vi "002_LinFlowChart.vi"(11 "Queue Ref In":T1={"UI"=refnum, "Message"=refnum, "Data"=refnum, "Caller"=refnum, "Name"="000 Common", "Data Path"=path "", "Class Path"=path "", "SubPanel"=refnum, "Project Name"="", "MNT"="", "Title"="", "Data Source"=refnum, "Queue List"={}, "VI"=refnum, "UE"=refnum}) -> ()   [LabVIEW 2020]
doc: "002_LinFlowChart.vi"
uses:
  Alin/QMH/000 Module Data Type.ctl
  Alin/QMH/Queue Message.ctl
  <vilib>/Utility/miscctls.llb/LVPoint32TypeDef.ctl
  <vilib>/Utility/miscctls.llb/LVBoundsTypeDef.ctl
  <vilib>/Utility/miscctls.llb/LVMapReplaceAction.ctl
  <vilib>/Utility/miscctls.llb/LVPositionTypeDef.ctl
  544e2817-58be-4d71-9deb-2b826c4f9655.vi
  <vilib>/Utility/config.llb/Read Key (String).vi
  <vilib>/Utility/file.llb/Read Delimited Spreadsheet (string).vi
  <vilib>/Utility/config.llb/Write Key (String).vi
  <vilib>/Utility/file.llb/Write Delimited Spreadsheet (string).vi
  <vilib>/Utility/config.llb/NI_LVConfig.lvlib
panel:
  in  "ShowLable":bool
  in  "WorkMode Edit":bool
  in  "Load Picture":bool
  in  "FlowChartEdit":bool
  in  "Picture Delete":bool
  in  "Picture Add":bool
  in  "Chart Select":u16(ring) items=["气路", "水路"]
  in  "LogRead":bool
  in  "Panel Show":bool
  in  "FlowChart":T2={"Bump 1"=FALSE, "Bump 2"=FALSE, "LMG 1"=FALSE, "LMG 2"=FALSE, "Data 1"="0", "Data 2"="0", "VValve 1"=FALSE, "HValve 1"=FALSE, "HValve 2"=FALSE, "VValve 2"=FALSE, "HFS 1"=FALSE, "VFS 1"=FALSE, "VFS 2"=FALSE, "HFS 2"=FALSE, "Data 3"="0", "Data 4"="0", "Data 5"="0", "Data 6"="0", "Data 7"="0", "Data 8"="0", "Data 9"="0", "Data 10"="0", "Data 11"="0", "Data 12"="0", "Data 13"="0", "Data 14"="0", "Data 15"="0", "Data 16"="0", "Data 17"="0", "Data 18"="0", "Data 19"="0", "Data 20"="0", "Data 21"="0", "Data 22"="0", "Data 23"="0", "Data 24"="0", "Data 25"="0", "Data 26"="0", "Data 27"="0", "Data 28"="0", "Data 29"="0", "Data 30"="0", "Data 31"="0", "Data 32"="0", "Data 33"="0", "Data 34"="0", "Data 35"="0", "Data 36"="0", "Data 37"="0", "Data 38"="0", "Data 39"="0", "Data 40"="0", "Data 41"="0", "Data 42"="0", "Data 43"="0", "Data 44"="0", "Data 45"="0", "Data 46"="0", "Data 47"="0", "Data 48"="0", "Data 49"="0", "Data 50"="0", "Data 51"="0", "Data 52"="0", "Data 53"="0", "Data 54"="0", "Data 55"="0", "Data 56"="0", "Data 57"="0", "Data 58"="0", "Data 59"="0", "Data 60"="0", "Data 61"="0", "Data 62"="0", "Data 63"="0", "Data 64"="0", "Data 65"="0", "Data 66"="0", "Data 67"="0", "Data 68"="0", "Data 69"="0", "Data 70"="0", "Data 71"="0", "Data 72"="0", "Data 73"="0", "Data 74"="0", "Data 75"="0", "Data 76"="0", "Data 77"="0", "Data 78"="0", "Data 79"="0", "Data 80"="0", "Data 81"="0", "Data 82"="0", "Data 83"="0", "Data 84"="0", "Data 85"="0", "Data 86"="0", "Data 87"="0", "Data 88"="0", "Data 89"="0", "Data 90"="0", "Data 91"="0", "Data 92"="0", "Data 93"="0", "Data 94"="0", "Data 95"="0", "Data 96"="0", "Data 97"="0", "Data 98"="0", "Data 99"="0", "Data 100"="0", "Data 101"="0", "Data 102"="0", "Data 103"="0", "Data 104"="0", "Data 105"="0", "Data 106"="0", "Data 107"="0", "Data 108"="0", "Data 109"="0", "Data 110"="0", "Data 111"="0", "Data 112"="0", "Data 113"="0", "Data 114"="0", "Data 115"="0", "Data 116"="0", "Data 117"="0", "Data 118"="0", "Data 119"="0", "Data 120"="0", "Data 121"="0", "Data 122"="0", "Data 123"="0", "Data 124"="0", "Data 125"="0", "Data 126"="0", "Data 127"="0", "Data 128"="0", "Data 129"="0", "Data 130"="0", "Data 131"="0", "Data 132"="0", "Data 133"="0", "Data 134"="0", "Data 135"="0", "Data 136"="0", "Data 137"="0", "Data 138"="0", "Data 139"="0", "Data 140"="0", "Data 141"="0", "Data 142"="0", "Data 143"="0", "Data 144"="0", "Data 145"="0", "Data 146"="0", "Data 147"="0", "Data 148"="0", "Data 149"="0", "Data 150"="0", "Data 151"="0", "Data 152"="0", "Data 153"="0", "Data 154"="0", "Data 155"="0", "Data 156"="0", "Data 157"="0", "Data 158"="0", "Data 159"="0", "Data 160"="0", "Data 161"="0", "Data 162"="0", "Data 163"="0", "Data 164"="0", "Data 165"="0", "Data 166"="0", "Data 167"="0", "Data 168"="0", "Data 169"="0", "Data 170"="0", "Data 171"="0", "Data 172"="0", "Data 173"="0", "Data 174"="0", "Data 175"="0", "Data 176"="0", "Data 177"="0", "Data 178"="0", "Data 179"="0", "Data 180"="0", "Data 181"="0", "Data 182"="0", "Data 183"="0", "Data 184"="0", "Data 185"="0", "Data 186"="0", "Data 187"="0", "Data 188"="0", "Data 189"="0", "Data 190"="0", "Data 191"="0", "Data 192"="0", "LMG 3"=FALSE, "LMG 4"=FALSE, "LMG 5"=FALSE, "LMG 6"=FALSE, "LMG 7"=FALSE, "LMG 8"=FALSE, "LMG 9"=FALSE, "LMG 10"=FALSE, "LMG 11"=FALSE, "LMG 12"=FALSE, "LMG 13"=FALSE, "LMG 14"=FALSE, "LMG 15"=FALSE, "LMG 16"=FALSE, "LMG 17"=FALSE, "LMG 18"=FALSE, "LMG 19"=FALSE, "LMG 20"=FALSE, "LMG 21"=FALSE, "LMG 22"=FALSE, "LMG 23"=FALSE, "LMG 24"=FALSE, "LMG 25"=FALSE, "LMG 26"=FALSE, "LMG 27"=FALSE, "LMG 28"=FALSE, "LMG 29"=FALSE, "LMG 30"=FALSE, "LMG 31"=FALSE, "LMG 32"=FALSE, "LMG 33"=FALSE, "LMG 34"=FALSE, "LMG 35"=FALSE, "LMG 36"=FALSE, "LMG 37"=FALSE, "LMG 38"=FALSE, "LMG 39"=FALSE, "LMG 40"=FALSE, "HValve 3"=FALSE, "HValve 4"=FALSE, "HValve 5"=FALSE, "HValve 6"=FALSE, "HValve 7"=FALSE, "HValve 8"=FALSE, "HValve 9"=FALSE, "HValve 10"=FALSE, "HValve 11"=FALSE, "HValve 12"=FALSE, "HValve 13"=FALSE, "HValve 14"=FALSE, "HValve 15"=FALSE, "HValve 16"=FALSE, "HValve 17"=FALSE, "HValve 18"=FALSE, "HValve 19"=FALSE, "HValve 20"=FALSE, "HValve 21"=FALSE, "HValve 22"=FALSE, "HValve 23"=FALSE, "HValve 24"=FALSE, "HValve 25"=FALSE, "HValve 26"=FALSE, "HValve 27"=FALSE, "HValve 28"=FALSE, "HValve 29"=FALSE, "HValve 30"=FALSE, "HValve 31"=FALSE, "HValve 32"=FALSE, "HValve 33"=FALSE, "HValve 34"=FALSE, "HValve 35"=FALSE, "HValve 36"=FALSE, "HValve 37"=FALSE, "HValve 38"=FALSE, "HValve 39"=FALSE, "HValve 40"=FALSE, "HValve 41"=FALSE, "HValve 42"=FALSE, "HValve 43"=FALSE, "HValve 44"=FALSE, "HValve 45"=FALSE, "HValve 46"=FALSE, "HValve 47"=FALSE, "HValve 48"=FALSE, "HValve 49"=FALSE, "HValve 50"=FALSE, "HValve 51"=FALSE, "HValve 52"=FALSE, "HValve 53"=FALSE, "HValve 54"=FALSE, "HValve 55"=FALSE, "HValve 56"=FALSE, "HValve 57"=FALSE, "HValve 58"=FALSE, "HValve 59"=FALSE, "HValve 60"=FALSE, "HValve 61"=FALSE, "HValve 62"=FALSE, "HValve 63"=FALSE, "HValve 64"=FALSE, "HValve 65"=FALSE, "HValve 66"=FALSE, "HValve 67"=FALSE, "HValve 68"=FALSE, "HValve 69"=FALSE, "HValve 70"=FALSE, "HValve 71"=FALSE, "HValve 72"=FALSE, "HValve 73"=FALSE, "HValve 74"=FALSE, "HValve 75"=FALSE, "HValve 76"=FALSE, "HValve 77"=FALSE, "HValve 78"=FALSE, "HValve 79"=FALSE, "HValve 80"=FALSE, "VValve 3"=FALSE, "VValve 4"=FALSE, "VValve 5"=FALSE, "VValve 6"=FALSE, "VValve 7"=FALSE, "VValve 8"=FALSE, "VValve 9"=FALSE, "VValve 10"=FALSE, "VValve 11"=FALSE, "VValve 12"=FALSE, "VValve 13"=FALSE, "VValve 14"=FALSE, "VValve 15"=FALSE, "VValve 16"=FALSE, "VValve 17"=FALSE, "VValve 18"=FALSE, "VValve 19"=FALSE, "VValve 20"=FALSE, "Bump 3"=FALSE, "Bump 4"=FALSE, "Bump 5"=FALSE, "Bump 6"=FALSE, "Bump 7"=FALSE, "Bump 8"=FALSE, "Bump 9"=FALSE, "Bump 10"=FALSE, "VFS 3"=FALSE, "VFS 4"=FALSE, "VFS 5"=FALSE, "VFS 6"=FALSE, "VFS 7"=FALSE, "VFS 8"=FALSE, "VFS 9"=FALSE, "VFS 10"=FALSE, "HFS 3"=FALSE, "HFS 4"=FALSE, "HFS 5"=FALSE, "HFS 6"=FALSE, "HFS 7"=FALSE, "HFS 8"=FALSE, "HFS 9"=FALSE, "HFS 10"=FALSE, "PRT 1"="0", "PRT 2"="0", "PRT 3"="0", "PRT 4"="0", "PRT 5"="0", "PRT 6"="0", "PRT 7"="0", "PRT 8"="0", "PRT 9"="0", "PRT 10"="0", "PRT 11"="0", "PRT 12"="0", "PRT 13"="0", "PRT 14"="0", "PRT 15"="0", "PRT 16"="0", "PRT 17"="0", "PRT 18"="0", "PRT 19"="0", "PRT 20"="0", "HVFS 1"=FALSE, "VVFS 1"=FALSE, "HVFS 2"=FALSE, "HVFS 3"=FALSE, "HVFS 4"=FALSE, "HVFS 5"=FALSE, "HVFS 6"=FALSE, "HVFS 7"=FALSE, "HVFS 8"=FALSE, "HVFS 9"=FALSE, "HVFS 10"=FALSE, "HVFS 11"=FALSE, "HVFS 12"=FALSE, "HVFS 13"=FALSE, "HVFS 14"=FALSE, "HVFS 15"=FALSE, "HVFS 16"=FALSE, "HVFS 17"=FALSE, "HVFS 18"=FALSE, "HVFS 19"=FALSE, "HVFS 20"=FALSE, "VVFS 2"=FALSE, "VVFS 3"=FALSE, "VVFS 4"=FALSE, "VVFS 5"=FALSE, "VVFS 6"=FALSE, "VVFS 7"=FALSE, "VVFS 8"=FALSE, "VVFS 9"=FALSE, "VVFS 10"=FALSE, "VVFS 11"=FALSE, "VVFS 12"=FALSE, "VVFS 13"=FALSE, "VVFS 14"=FALSE, "VVFS 15"=FALSE, "VVFS 16"=FALSE, "VVFS 17"=FALSE, "VVFS 18"=FALSE, "VVFS 19"=FALSE, "VVFS 20"=FALSE, "NHVFS 100"=FALSE, "NVFS 100"=FALSE, "NHFS 100"=FALSE, "NHVFS 101"=FALSE, "NVFS 101"=FALSE, "NHFS 101"=FALSE, "NHVFS 102"=FALSE, "NVFS 102"=FALSE, "NHFS 102"=FALSE, "NHVFS 103"=FALSE, "NVFS 103"=FALSE, "NHFS 103"=FALSE, "NHVFS 104"=FALSE, "NVFS 104"=FALSE, "NHFS 104"=FALSE, "NHVFS 105"=FALSE, "NVFS 105"=FALSE, "NHFS 105"=FALSE, "NHVFS 106"=FALSE, "NVFS 106"=FALSE, "NHFS 106"=FALSE, "NHVFS 107"=FALSE, "NVFS 107"=FALSE, "NHFS 107"=FALSE, "NHVFS 108"=FALSE, "NVFS 108"=FALSE, "NHFS 108"=FALSE, "NHVFS 109"=FALSE, "NVFS 109"=FALSE, "NHFS 109"=FALSE}
  out "Picture":picture
  out "Tips":string
  in  "Decimal":u16=1 max=6
  in  "Horizontal scroll bar":bool caption="H"
  in  "Vertical scroll bar":bool caption="V"
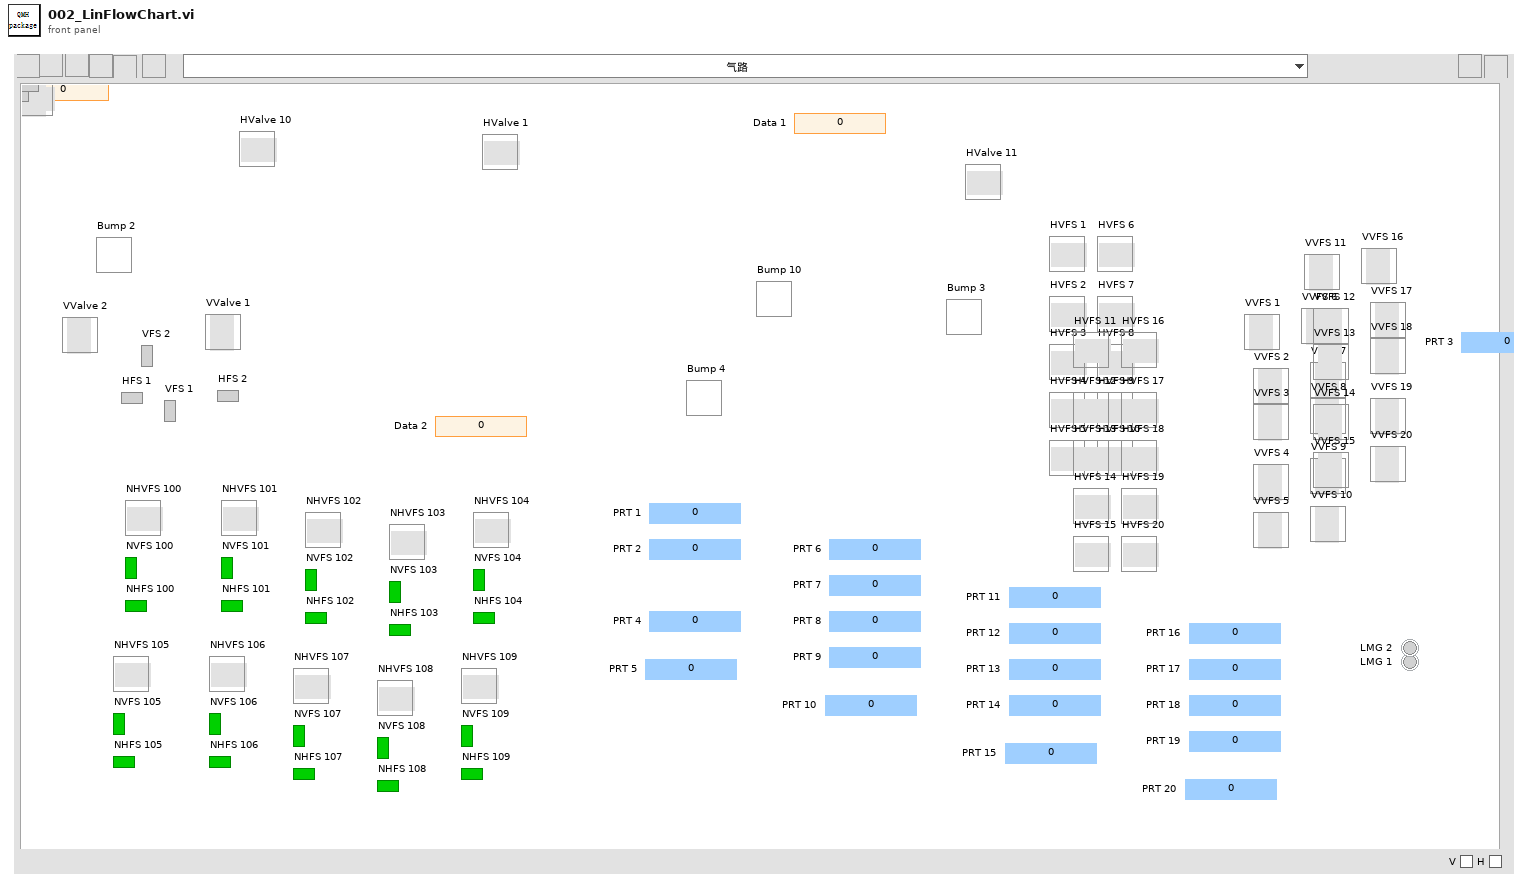
[diagram p1: front panel]
types:
  T1 = typedef "000 Module Data Type.ctl" = cluster{"UI":refnum<queue>, "Message":refnum<queue>, "Data":refnum<queue>, "Caller":refnum<queue>, "Name":string, "Data Path":path, "Class Path":path, "SubPanel":refnum<vi>, "Project Name":string, "MNT":string, "Title":string, "Data Source":refnum<queue>, "Queue List":map{string, refnum<queue>}, "VI":refnum<vi>, "UE":refnum<user-event>}
  T2 = cluster{"Bump 1":bool, "Bump 2":bool, "LMG 1":bool, "LMG 2":bool, "Data 1":string, "Data 2":string, "VValve 1":bool, "HValve 1":bool, "HValve 2":bool, "VValve 2":bool, "HFS 1":bool, "VFS 1":bool, "VFS 2":bool, "HFS 2":bool, "Data 3":string, "Data 4":string, "Data 5":string, "Data 6":string, "Data 7":string, "Data 8":string, "Data 9":string, "Data 10":string, "Data 11":string, "Data 12":string, "Data 13":string, "Data 14":string, "Data 15":string, "Data 16":string, "Data 17":string, "Data 18":string, "Data 19":string, "Data 20":string, "Data 21":string, "Data 22":string, "Data 23":string, "Data 24":string, "Data 25":string, "Data 26":string, "Data 27":string, "Data 28":string, "Data 29":string, "Data 30":string, "Data 31":string, "Data 32":string, "Data 33":string, "Data 34":string, "Data 35":string, "Data 36":string, "Data 37":string, "Data 38":string, "Data 39":string, "Data 40":string, "Data 41":string, "Data 42":string, "Data 43":string, "Data 44":string, "Data 45":string, "Data 46":string, "Data 47":string, "Data 48":string, "Data 49":string, "Data 50":string, "Data 51":string, "Data 52":string, "Data 53":string, "Data 54":string, "Data 55":string, "Data 56":string, "Data 57":string, "Data 58":string, "Data 59":string, "Data 60":string, "Data 61":string, "Data 62":string, "Data 63":string, "Data 64":string, "Data 65":string, "Data 66":string, "Data 67":string, "Data 68":string, "Data 69":string, "Data 70":string, "Data 71":string, "Data 72":string, "Data 73":string, "Data 74":string, "Data 75":string, "Data 76":string, "Data 77":string, "Data 78":string, "Data 79":string, "Data 80":string, "Data 81":string, "Data 82":string, "Data 83":string, "Data 84":string, "Data 85":string, "Data 86":string, "Data 87":string, "Data 88":string, "Data 89":string, "Data 90":string, "Data 91":string, "Data 92":string, "Data 93":string, "Data 94":string, "Data 95":string, "Data 96":string, "Data 97":string, "Data 98":string, "Data 99":string, "Data 100":string, "Data 101":string, "Data 102":string, "Data 103":string, "Data 104":string, "Data 105":string, "Data 106":string, "Data 107":string, "Data 108":string, "Data 109":string, "Data 110":string, "Data 111":string, "Data 112":string, "Data 113":string, "Data 114":string, "Data 115":string, "Data 116":string, "Data 117":string, "Data 118":string, "Data 119":string, "Data 120":string, "Data 121":string, "Data 122":string, "Data 123":string, "Data 124":string, "Data 125":string, "Data 126":string, "Data 127":string, "Data 128":string, "Data 129":string, "Data 130":string, "Data 131":string, "Data 132":string, "Data 133":string, "Data 134":string, "Data 135":string, "Data 136":string, "Data 137":string, "Data 138":string, "Data 139":string, "Data 140":string, "Data 141":string, "Data 142":string, "Data 143":string, "Data 144":string, "Data 145":string, "Data 146":string, "Data 147":string, "Data 148":string, "Data 149":string, "Data 150":string, "Data 151":string, "Data 152":string, "Data 153":string, "Data 154":string, "Data 155":string, "Data 156":string, "Data 157":string, "Data 158":string, "Data 159":string, "Data 160":string, "Data 161":string, "Data 162":string, "Data 163":string, "Data 164":string, "Data 165":string, "Data 166":string, "Data 167":string, "Data 168":string, "Data 169":string, "Data 170":string, "Data 171":string, "Data 172":string, "Data 173":string, "Data 174":string, "Data 175":string, "Data 176":string, "Data 177":string, "Data 178":string, "Data 179":string, "Data 180":string, "Data 181":string, "Data 182":string, "Data 183":string, "Data 184":string, "Data 185":string, "Data 186":string, "Data 187":string, "Data 188":string, "Data 189":string, "Data 190":string, "Data 191":string, "Data 192":string, "LMG 3":bool, "LMG 4":bool, "LMG 5":bool, "LMG 6":bool, "LMG 7":bool, "LMG 8":bool, "LMG 9":bool, "LMG 10":bool, "LMG 11":bool, "LMG 12":bool, "LMG 13":bool, "LMG 14":bool, "LMG 15":bool, "LMG 16":bool, "LMG 17":bool, "LMG 18":bool, "LMG 19":bool, "LMG 20":bool, "LMG 21":bool, "LMG 22":bool, "LMG 23":bool, "LMG 24":bool, "LMG 25":bool, "LMG 26":bool, "LMG 27":bool, "LMG 28":bool, "LMG 29":bool, "LMG 30":bool, "LMG 31":bool, "LMG 32":bool, "LMG 33":bool, "LMG 34":bool, "LMG 35":bool, "LMG 36":bool, "LMG 37":bool, "LMG 38":bool, "LMG 39":bool, "LMG 40":bool, "HValve 3":bool, "HValve 4":bool, "HValve 5":bool, "HValve 6":bool, "HValve 7":bool, "HValve 8":bool, "HValve 9":bool, "HValve 10":bool, "HValve 11":bool, "HValve 12":bool, "HValve 13":bool, "HValve 14":bool, "HValve 15":bool, "HValve 16":bool, "HValve 17":bool, "HValve 18":bool, "HValve 19":bool, "HValve 20":bool, "HValve 21":bool, "HValve 22":bool, "HValve 23":bool, "HValve 24":bool, "HValve 25":bool, "HValve 26":bool, "HValve 27":bool, "HValve 28":bool, "HValve 29":bool, "HValve 30":bool, "HValve 31":bool, "HValve 32":bool, "HValve 33":bool, "HValve 34":bool, "HValve 35":bool, "HValve 36":bool, "HValve 37":bool, "HValve 38":bool, "HValve 39":bool, "HValve 40":bool, "HValve 41":bool, "HValve 42":bool, "HValve 43":bool, "HValve 44":bool, "HValve 45":bool, "HValve 46":bool, "HValve 47":bool, "HValve 48":bool, "HValve 49":bool, "HValve 50":bool, "HValve 51":bool, "HValve 52":bool, "HValve 53":bool, "HValve 54":bool, "HValve 55":bool, "HValve 56":bool, "HValve 57":bool, "HValve 58":bool, "HValve 59":bool, "HValve 60":bool, "HValve 61":bool, "HValve 62":bool, "HValve 63":bool, "HValve 64":bool, "HValve 65":bool, "HValve 66":bool, "HValve 67":bool, "HValve 68":bool, "HValve 69":bool, "HValve 70":bool, "HValve 71":bool, "HValve 72":bool, "HValve 73":bool, "HValve 74":bool, "HValve 75":bool, "HValve 76":bool, "HValve 77":bool, "HValve 78":bool, "HValve 79":bool, "HValve 80":bool, "VValve 3":bool, "VValve 4":bool, "VValve 5":bool, "VValve 6":bool, "VValve 7":bool, "VValve 8":bool, "VValve 9":bool, "VValve 10":bool, "VValve 11":bool, "VValve 12":bool, "VValve 13":bool, "VValve 14":bool, "VValve 15":bool, "VValve 16":bool, "VValve 17":bool, "VValve 18":bool, "VValve 19":bool, "VValve 20":bool, "Bump 3":bool, "Bump 4":bool, "Bump 5":bool, "Bump 6":bool, "Bump 7":bool, "Bump 8":bool, "Bump 9":bool, "Bump 10":bool, "VFS 3":bool, "VFS 4":bool, "VFS 5":bool, "VFS 6":bool, "VFS 7":bool, "VFS 8":bool, "VFS 9":bool, "VFS 10":bool, "HFS 3":bool, "HFS 4":bool, "HFS 5":bool, "HFS 6":bool, "HFS 7":bool, "HFS 8":bool, "HFS 9":bool, "HFS 10":bool, "PRT 1":string, "PRT 2":string, "PRT 3":string, "PRT 4":string, "PRT 5":string, "PRT 6":string, "PRT 7":string, "PRT 8":string, "PRT 9":string, "PRT 10":string, "PRT 11":string, "PRT 12":string, "PRT 13":string, "PRT 14":string, "PRT 15":string, "PRT 16":string, "PRT 17":string, "PRT 18":string, "PRT 19":string, "PRT 20":string, "HVFS 1":bool, "VVFS 1":bool, "HVFS 2":bool, "HVFS 3":bool, "HVFS 4":bool, "HVFS 5":bool, "HVFS 6":bool, "HVFS 7":bool, "HVFS 8":bool, "HVFS 9":bool, "HVFS 10":bool, "HVFS 11":bool, "HVFS 12":bool, "HVFS 13":bool, "HVFS 14":bool, "HVFS 15":bool, "HVFS 16":bool, "HVFS 17":bool, "HVFS 18":bool, "HVFS 19":bool, "HVFS 20":bool, "VVFS 2":bool, "VVFS 3":bool, "VVFS 4":bool, "VVFS 5":bool, "VVFS 6":bool, "VVFS 7":bool, "VVFS 8":bool, "VVFS 9":bool, "VVFS 10":bool, "VVFS 11":bool, "VVFS 12":bool, "VVFS 13":bool, "VVFS 14":bool, "VVFS 15":bool, "VVFS 16":bool, "VVFS 17":bool, "VVFS 18":bool, "VVFS 19":bool, "VVFS 20":bool, "NHVFS 100":bool, "NVFS 100":bool, "NHFS 100":bool, "NHVFS 101":bool, "NVFS 101":bool, "NHFS 101":bool, "NHVFS 102":bool, "NVFS 102":bool, "NHFS 102":bool, "NHVFS 103":bool, "NVFS 103":bool, "NHFS 103":bool, "NHVFS 104":bool, "NVFS 104":bool, "NHFS 104":bool, "NHVFS 105":bool, "NVFS 105":bool, "NHFS 105":bool, "NHVFS 106":bool, "NVFS 106":bool, "NHFS 106":bool, "NHVFS 107":bool, "NVFS 107":bool, "NHFS 107":bool, "NHVFS 108":bool, "NVFS 108":bool, "NHFS 108":bool, "NHVFS 109":bool, "NVFS 109":bool, "NHFS 109":bool}
  T3 = typedef "LVBoundsTypeDef.ctl" = cluster{"Width":u32, "Height":u32}
  T4 = cluster{"Queue":T1, "Property":map{string, cluster{"Type":string, "Control":string, "Name":string, "ID":string, "Show":bool, "Top":i32, "Left":i32, "Ref":refnum<vi>}}, "Type":map{string, map{string, refnum<vi>}}, "UE":refnum<user-event>, "Area":T3, "Panel":refnum<vi>, "Bar?":bool, "PictureList":string[], "Picture":refnum<vi>, "CPicture":string, "Chart Select":refnum<vi>, "WorkMode":cluster{"Mode":string, "Data":string, "Mode?":bool}}
  T5 = cluster{"Queue":T1, "Delay":cluster{"Count Time(ms)":u32, "Delay Time(ms)":u32, "Next":string}, "Panel":refnum<vi>, "Property":map{string, cluster{"Type":string, "Control":string, "Name":string, "ID":string, "Show":bool, "Top":i32, "Left":i32, "Ref":refnum<vi>}}, "File":path, "CPicture":string, "Mode":cluster{"Mode":string, "Data":string}}
  T6 = typedef "LVPoint32TypeDef.ctl" = cluster{"Horizontal":i32, "Vertical":i32}
  T7 = cluster{"Object":refnum<vi>, "Init":T6, "ON?":bool, "Type":map{string, map{string, refnum<vi>}}}
  T8 = enum8{"Enabled", "Disabled", "Disabled and Grayed Out"}
  T9 = typedef "eventvkey.ctl" = enum16{"ASCII", "Enter", "Return", "Shift", "Ctrl", "Alt", "Cmd", "Opt", "Caps", "NumLock", "Clear", "Break", "Up", "Down", "Left", "Right", "Insert", "Delete", "Home", "End", "PageUp", "PageDown", "Escape", "Help", "Pause", "ScrollLock", "F1", "F2", "F3", "F4", "F5", "F6", "F7", "F8", "F9", "F10", "F11", "F12", "F13", "F14", "F15", "F16", "F17", "F18", "F19", "F20", "F21", "F22", "F23", "F24", "Play", "VolumeUp", "VolumeDown", "Mute", "Two Byte Char"}
  T10 = cluster{"Shift":bool, "Ctrl":bool, "Alt":bool, "Cmd":bool, "Opt":bool}
  T11 = typedef "LVPositionTypeDef.ctl" = cluster{"Left":i32, "Top":i32}
  T12 = typedef "LVMapReplaceAction.ctl" = enum32{"Modify Entry only if found", "Add or Modify Entry", "Delete Entry"}
  T13 = map{string, cluster{"Type":string, "Control":string, "Name":string, "ID":string, "Show":bool, "Top":i32, "Left":i32, "Ref":refnum<vi>}}
  T14 = cluster{"Type":string, "Control":string, "Name":string, "ID":string, "Show":bool, "Top":i32, "Left":i32, "Ref":refnum<vi>}
  T15 = typedef "NI_LVConfig.lvlib/Config Data RefNum.ctl" = refnum<k1>
  T16 = typedef "SDQ Data Type.ctl" = cluster{"CAN Length":string, "CAN Name":string, "CAN ID":string, "CAN Type":string, "Test Item":string, "Byte Order":string, "Instruction":string, "Control Type":string, "Group":string, "Offset":dbl, "Coefficient":dbl, "Write Enable":bool, "Lable Type":string, "Key?":string, "Set Value":string, "Upper":dbl, "Lower":dbl, "Unit":string, "Formula":string, "Test Item Type":string, "Length":i32, "Address":string, "Name":string, "Identifier":string, "Data Type":string, "Enumerate?":string, "Enumerate List":string, "Data":string, "Source":string}
  T17 = enum16{"Always On", "Always Off", "Off While Running"}
  T18 = typedef "imagedata.ctl" = cluster{"image type":i32, "image depth":i32, "image":u8[], "mask":u8[], "colors":u32[], "Rectangle":cluster{"left":i16, "top":i16, "right":i16, "bottom":i16}}
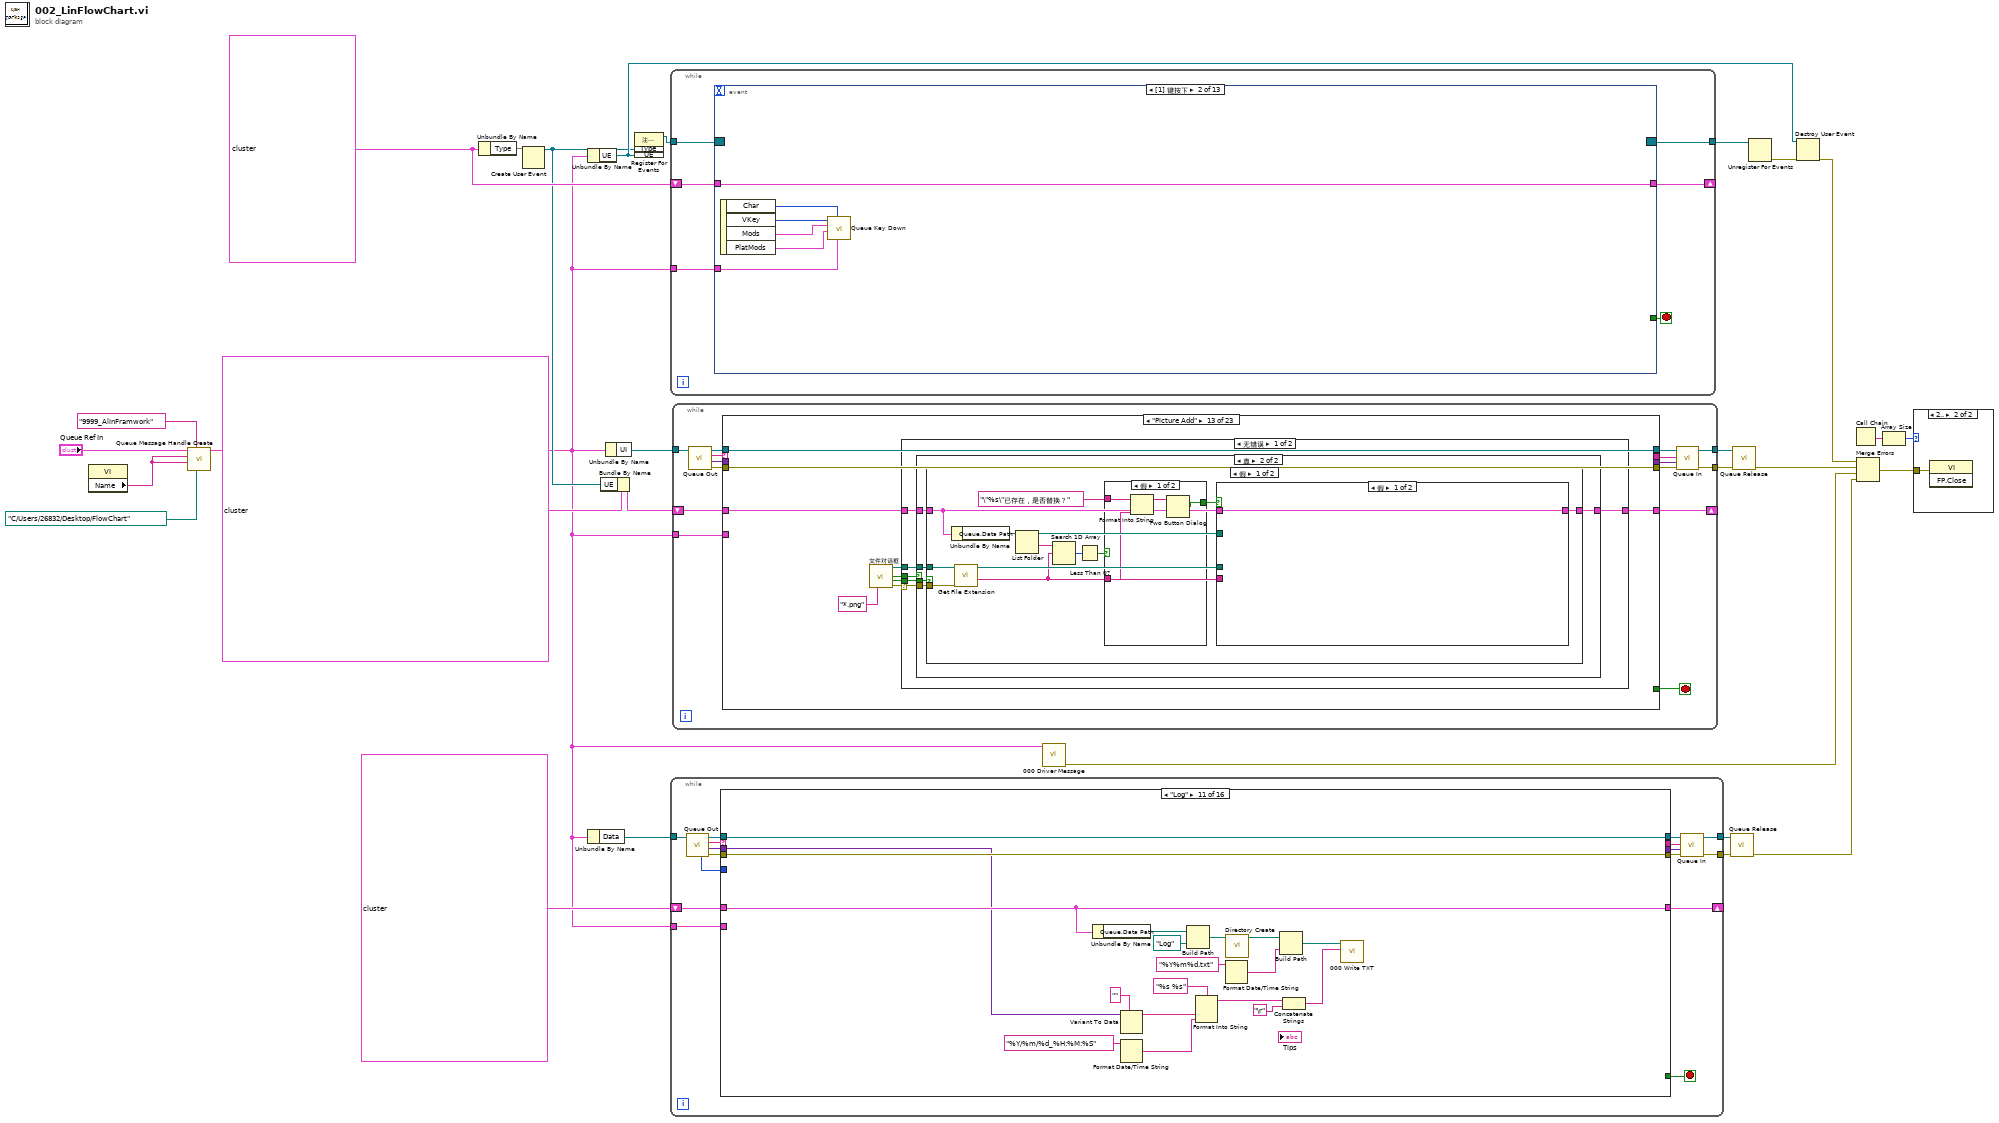
[diagram p0: block diagram]
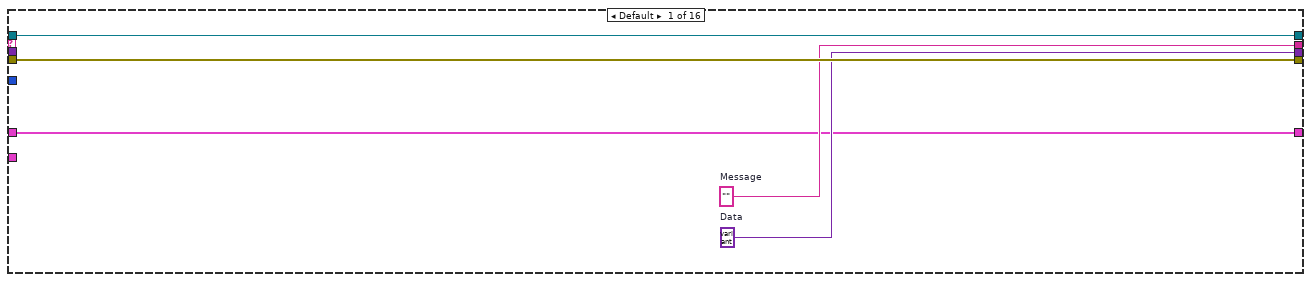
[diagram p2: hidden frame]
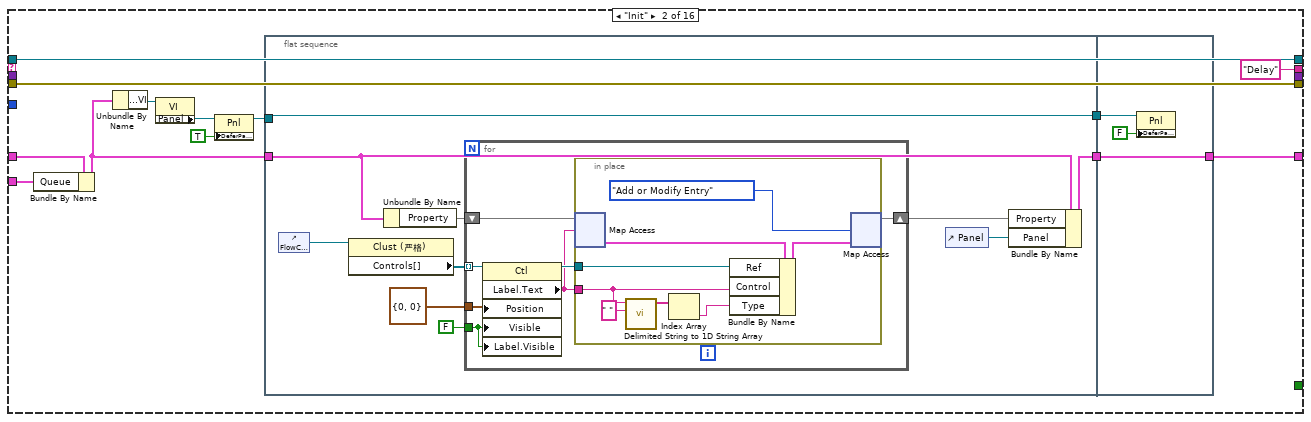
[diagram p3: hidden frame]
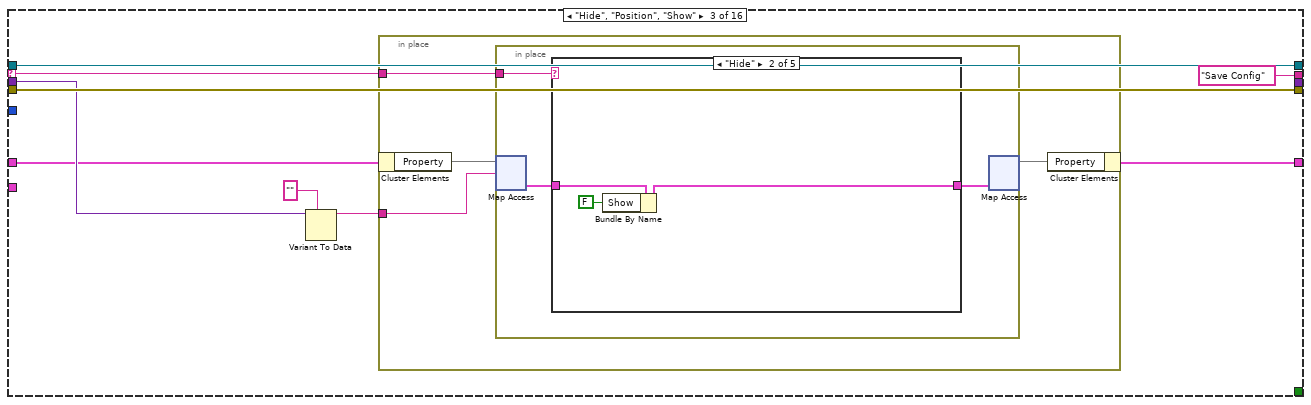
[diagram p4: hidden frame]
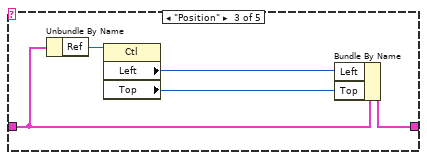
[diagram p6: hidden frame]
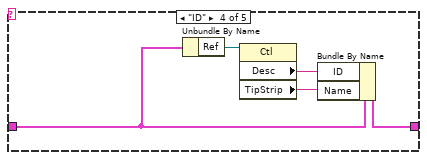
[diagram p7: hidden frame]
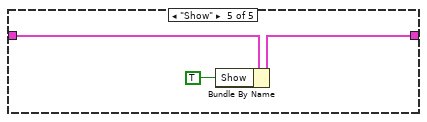
[diagram p8: hidden frame]
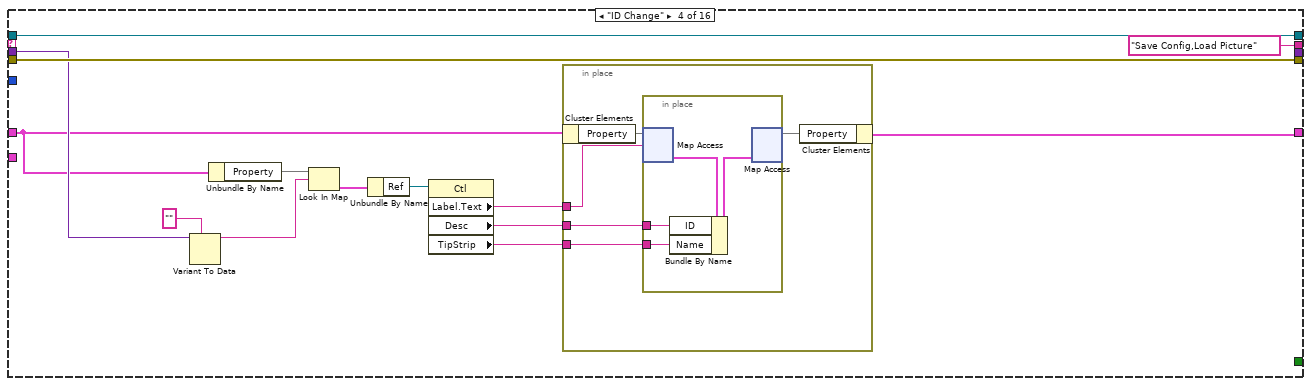
[diagram p9: hidden frame]
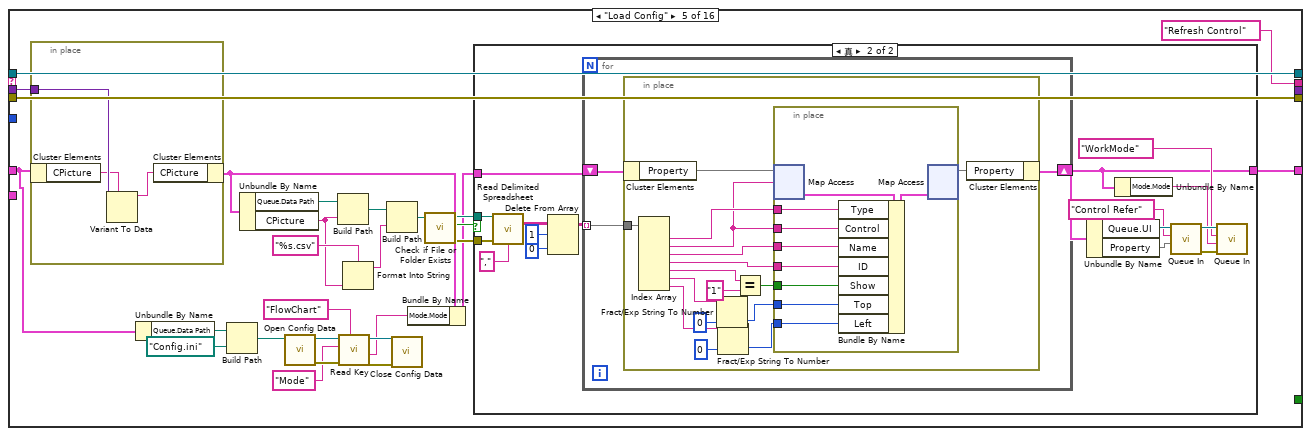
[diagram p10: hidden frame]
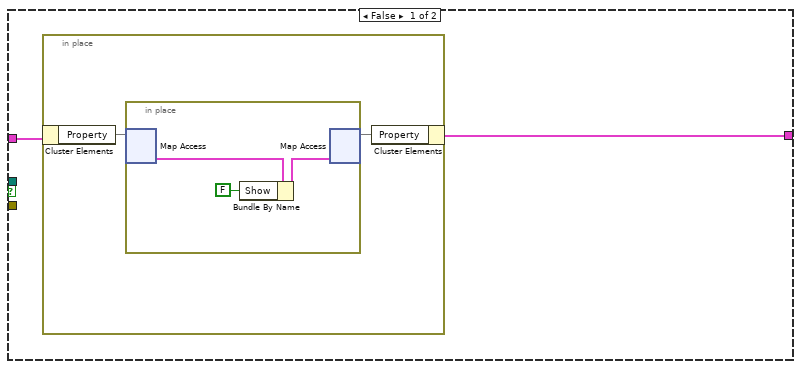
[diagram p11: hidden frame]
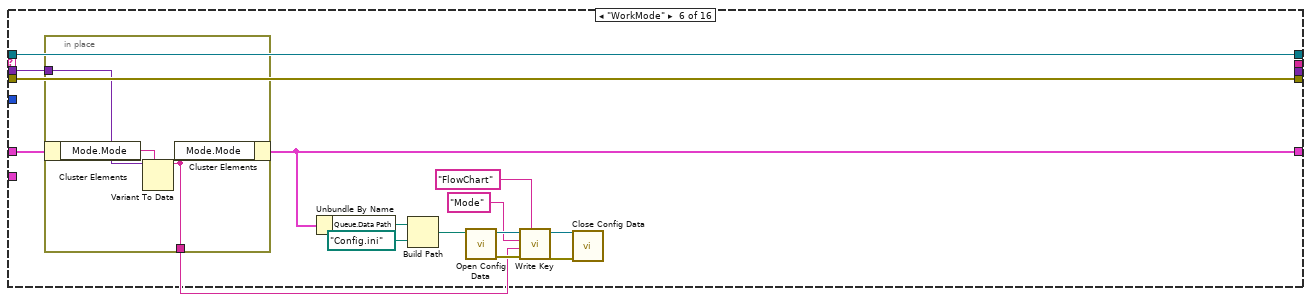
[diagram p12: hidden frame]
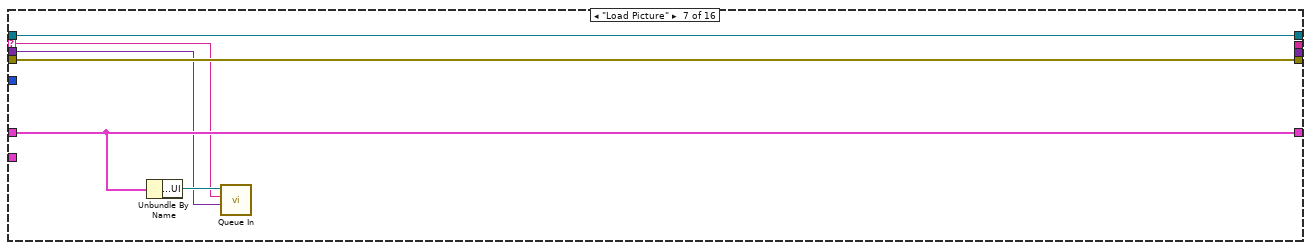
[diagram p13: hidden frame]
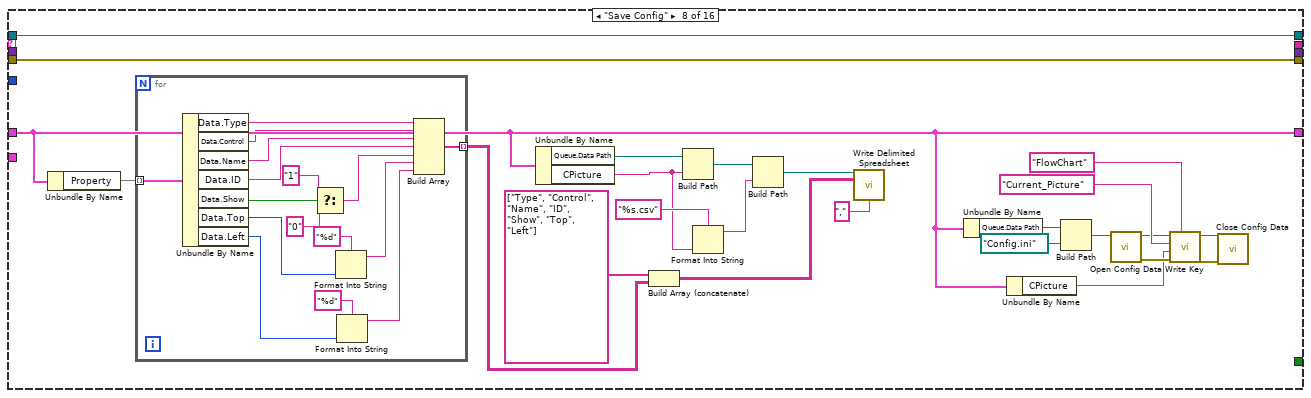
[diagram p14: hidden frame]
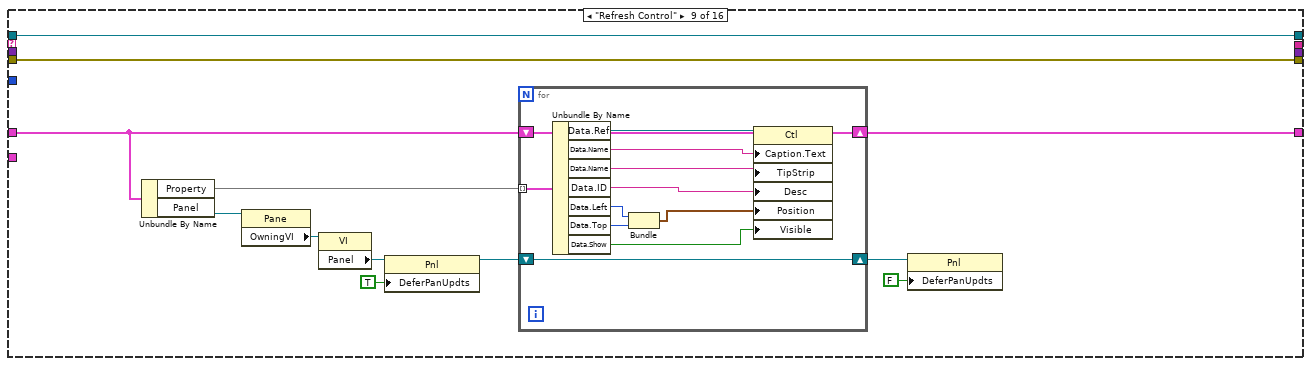
[diagram p15: hidden frame]
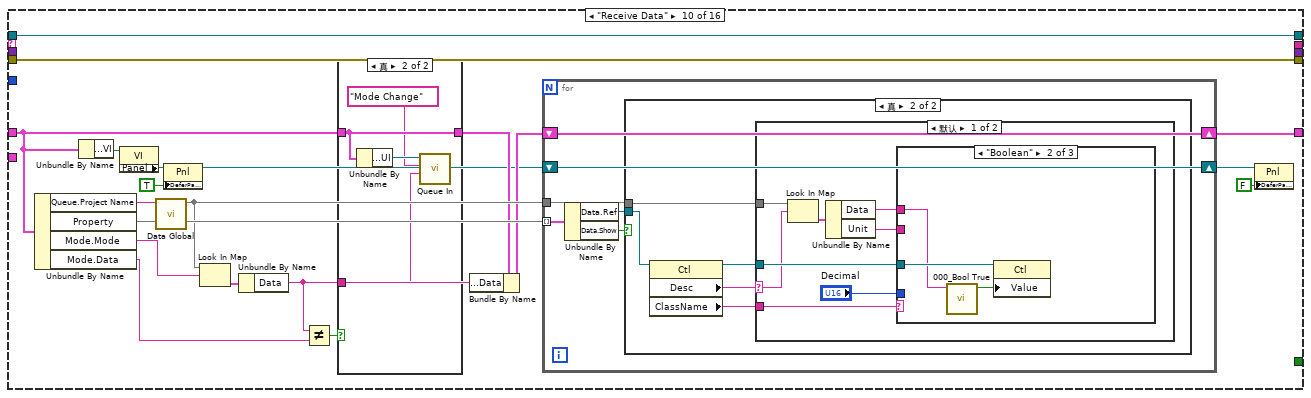
[diagram p16: hidden frame]
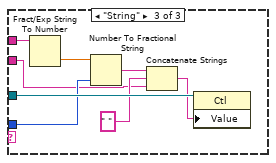
[diagram p20: hidden frame]
diagram:
  w7 = T7 {"Object"=refnum, "Init"={"Horizontal"=0, "Vertical"=0}, "ON?"=FALSE, "Type"={}}
  n1 = property class="VI"() -> ("Name"=w2:string)  [unwired: 2 in, 2 out]
  n2 = call "Queue Message Handle Create.vi"("Data Path"=path "C:/Users/26832/Desktop/FlowChart", "Project Name"="9999_AlinFramwork", "Name"=w2, "Title"=w2, "Queue Ref In"="Queue Ref In") -> ("Queue Ref Out"=w3:T1)  [unwired: 5 in, 1 out]
  n3 = Unbundle By Name(w7) -> ("Type"=w6:map{string, map{string, refnum<vi>}})
  n4 = Create User Event(user event datatype=w6) -> (user event=w4:refnum<user-event>)  [unwired: 1 in, 1 out]
  n5 = Unbundle By Name(w3) -> ("UE"=w12:refnum<user-event>)
  n6 = Unbundle By Name(w3) -> ("Data"=w15:refnum<queue>)
  n7 = Bundle By Name(cluster=T4 {"Queue"={"UI"=refnum, "Message"=refnum, "Data"=refnum, "Caller"=refnum, "Name"="000 Common", "Data Path"=path "", "Class Path"=path "", "SubPanel"=refnum, "Project Name"="", "MNT"="", "Title"="", "Data Source"=refnum, "Queue List"={}, "VI"=refnum, "UE"=refnum}, "Property"={}, "Type"={}, "UE"=refnum, "Area"={"Width"=0, "Height"=0}, "Panel"=refnum, "Bar?"=FALSE, "PictureList"=[], "Picture"=refnum, "CPicture"="", "Chart Select"=refnum, "WorkMode"={"Mode"="", "Data"="", "Mode?"=FALSE}}, "UE"=w4) -> (w5:T4)
  n8 = Unbundle By Name(w3) -> ("UI"=w23:refnum<queue>)
  n9 = register-events(w4, w12) -> (reference out=w28:refnum<event-registration>)  [unwired: 2 in, 1 out]
  n10 = while {
    tunnel: w28 -> [w34]
    tunnel: [w32] -> w27
    tunnel: w3 -> [w31]
    shift-right: [w29] -> _
    shift-left: w7 -> [w30]
    stop <- w33 stop-if-true
    n11 = event shown="[1] 键按下" {
      selector: w34 -> [_ _ _ _ _ _ _ _ _ _ _ _ _]
      dyn-events: [_ _ _ _ _ _ _ _ _ _ _ _ _] -> w32
      timeout: _ -> [_ _ _ _ _ _ _ _ _ _ _ _ _]
      tunnel: [_ _ _ _ _ _ _ w129 _ _ _ _ _] -> w33
      tunnel: w31 -> [_ w39 w44 w94 _ _ w116 _ w135 w147 w152 w156 w161]
      tunnel: w30 -> [w35 w41 w55 w97 w100 w103 w119 w128 w132 w148 w153 w158 w163]
      tunnel: [w35 w41 w51 w97 w99 w102 w121 w128 w132 w148 w153 w158 w163] -> w29
      event Timeout {
        n12 = event-data() -> ()  [unwired: 1 in, 1 out]
      }
      event Key Down {
        n13 = event-data() -> ("Char"=w40:i16, "VKey"=w38:T9, "Mods"=w37:cluster{"Num Pad":bool, "Menu Key":bool}, "PlatMods"=w36:T10)  [unwired: 1 in]
        n14 = call "Queue Key Down.vi"("Queue Ref Out"=w39, "C"=w40, "Platform Key"=w36, "Group Key"=w37, "V Key"=w38) -> ()  [unwired: 6 in, 1 out]
      }
      event "FlowChart", "FlowChart.Bump 1", "FlowChart.Bump 2", "FlowChart.LMG 1", "FlowChart.LMG 2", "FlowChart.Data 1", "FlowChart.Data 2", "FlowChart.HFS 1", "FlowChart.VFS 1", "FlowChart.VFS 2", "FlowChart.HFS 2", "FlowChart.VValve 2", "FlowChart.HValve 2", "FlowChart.HValve 1", "FlowChart.VValve 1", "FlowChart.Data 3", "FlowChart.Data 4", "FlowChart.Data 5", "FlowChart.Data 6", "FlowChart.Data 7", "FlowChart.Data 8", "FlowChart.Data 9", "FlowChart.Data 10", "FlowChart.Data 11", "FlowChart.Data 12", "FlowChart.Data 13", "FlowChart.Data 14", "FlowChart.Data 15", "FlowChart.Data 16", "FlowChart.Data 17", "FlowChart.Data 18", "FlowChart.Data 19", "FlowChart.Data 20", "FlowChart.Data 21", "FlowChart.Data 22", "FlowChart.Data 23", "FlowChart.Data 24", "FlowChart.Data 25", "FlowChart.Data 26", "FlowChart.Data 27", "FlowChart.Data 28", "FlowChart.Data 29", "FlowChart.Data 30", "FlowChart.Data 31", "FlowChart.Data 32", "FlowChart.Data 33", "FlowChart.Data 34", "FlowChart.Data 35", "FlowChart.Data 36", "FlowChart.Data 37", "FlowChart.Data 38", "FlowChart.Data 39", "FlowChart.Data 40", "FlowChart.Data 41", "FlowChart.Data 42", "FlowChart.Data 43", "FlowChart.Data 44", "FlowChart.Data 45", "FlowChart.Data 46", "FlowChart.Data 47", "FlowChart.Data 48", "FlowChart.Data 49", "FlowChart.Data 50", "FlowChart.Data 51", "FlowChart.Data 52", "FlowChart.Data 53", "FlowChart.Data 54", "FlowChart.Data 55", "FlowChart.Data 56", "FlowChart.Data 57", "FlowChart.Data 58", "FlowChart.Data 59", "FlowChart.Data 60", "FlowChart.Data 61", "FlowChart.Data 62", "FlowChart.Data 63", "FlowChart.Data 64", "FlowChart.Data 65", "FlowChart.Data 66", "FlowChart.Data 67", "FlowChart.Data 68", "FlowChart.Data 69", "FlowChart.Data 70", "FlowChart.Data 71", "FlowChart.Data 72", "FlowChart.Data 73", "FlowChart.Data 74", "FlowChart.Data 75", "FlowChart.Data 76", "FlowChart.Data 77", "FlowChart.Data 78", "FlowChart.Data 79", "FlowChart.Data 80", "FlowChart.Data 81", "FlowChart.Data 82", "FlowChart.Data 83", "FlowChart.Data 84", "FlowChart.Data 85", "FlowChart.Data 86", "FlowChart.Data 87", "FlowChart.Data 88", "FlowChart.Data 89", "FlowChart.Data 90", "FlowChart.Data 91", "FlowChart.Data 92", "FlowChart.Data 93", "FlowChart.Data 94", "FlowChart.Data 95", "FlowChart.Data 96", "FlowChart.Data 97", "FlowChart.Data 98", "FlowChart.Data 99", "FlowChart.Data 100", "FlowChart.Data 101", "FlowChart.Data 102", "FlowChart.Data 103", "FlowChart.Data 104", "FlowChart.Data 105", "FlowChart.Data 106", "FlowChart.Data 107", "FlowChart.Data 108", "FlowChart.Data 109", "FlowChart.Data 110", "FlowChart.Data 111", "FlowChart.Data 112", "FlowChart.Data 113", "FlowChart.Data 114", "FlowChart.Data 115", "FlowChart.Data 116", "FlowChart.Data 117", "FlowChart.Data 118", "FlowChart.Data 119", "FlowChart.Data 120", "FlowChart.Data 121", "FlowChart.Data 122", "FlowChart.Data 123", "FlowChart.Data 124", "FlowChart.Data 125", "FlowChart.Data 126", "FlowChart.Data 127", "FlowChart.Data 128", "FlowChart.Data 129", "FlowChart.Data 130", "FlowChart.Data 131", "FlowChart.Data 132", "FlowChart.Data 133", "FlowChart.Data 134", "FlowChart.Data 135", "FlowChart.Data 136", "FlowChart.Data 137", "FlowChart.Data 138", "FlowChart.Data 139", "FlowChart.Data 140", "FlowChart.Data 141", "FlowChart.Data 142", "FlowChart.Data 143", "FlowChart.Data 144", "FlowChart.Data 145", "FlowChart.Data 146", "FlowChart.Data 147", "FlowChart.Data 148", "FlowChart.Data 149", "FlowChart.Data 150", "FlowChart.Data 151", "FlowChart.Data 152", "FlowChart.Data 153", "FlowChart.Data 154", "FlowChart.Data 155", "FlowChart.Data 156", "FlowChart.Data 157", "FlowChart.Data 158", "FlowChart.Data 159", "FlowChart.Data 160", "FlowChart.Data 161", "FlowChart.Data 162", "FlowChart.Data 163", "FlowChart.Data 164", "FlowChart.Data 165", "FlowChart.Data 166", "FlowChart.Data 167", "FlowChart.Data 168", "FlowChart.Data 169", "FlowChart.Data 170", "FlowChart.Data 171", "FlowChart.Data 172", "FlowChart.Data 173", "FlowChart.Data 174", "FlowChart.Data 175", "FlowChart.Data 176", "FlowChart.Data 177", "FlowChart.Data 178", "FlowChart.Data 179", "FlowChart.Data 180", "FlowChart.Data 181", "FlowChart.Data 182", "FlowChart.Data 183", "FlowChart.Data 184", "FlowChart.Data 185", "FlowChart.Data 186", "FlowChart.Data 187", "FlowChart.Data 188", "FlowChart.Data 189", "FlowChart.Data 190", "FlowChart.Data 191", "FlowChart.Data 192", "FlowChart.LMG 3", "FlowChart.LMG 4", "FlowChart.LMG 5", "FlowChart.LMG 6", "FlowChart.LMG 7", "FlowChart.LMG 8", "FlowChart.LMG 9", "FlowChart.LMG 10", "FlowChart.LMG 11", "FlowChart.LMG 12", "FlowChart.LMG 13", "FlowChart.LMG 14", "FlowChart.LMG 15", "FlowChart.LMG 16", "FlowChart.LMG 17", "FlowChart.LMG 18", "FlowChart.LMG 19", "FlowChart.LMG 20", "FlowChart.LMG 21", "FlowChart.LMG 22", "FlowChart.LMG 23", "FlowChart.LMG 24", "FlowChart.LMG 25", "FlowChart.LMG 26", "FlowChart.LMG 27", "FlowChart.LMG 28", "FlowChart.LMG 29", "FlowChart.LMG 30", "FlowChart.LMG 31", "FlowChart.LMG 32", "FlowChart.LMG 33", "FlowChart.LMG 34", "FlowChart.LMG 35", "FlowChart.LMG 36", "FlowChart.LMG 37", "FlowChart.LMG 38", "FlowChart.LMG 39", "FlowChart.LMG 40", "FlowChart.HValve 3", "FlowChart.HValve 4", "FlowChart.HValve 5", "FlowChart.HValve 6", "FlowChart.HValve 7", "FlowChart.HValve 8", "FlowChart.HValve 9", "FlowChart.HValve 10", "FlowChart.HValve 11", "FlowChart.HValve 12", "FlowChart.HValve 13", "FlowChart.HValve 14", "FlowChart.HValve 15", "FlowChart.HValve 16", "FlowChart.HValve 17", "FlowChart.HValve 18", "FlowChart.HValve 19", "FlowChart.HValve 20", "FlowChart.HValve 21", "FlowChart.HValve 22", "FlowChart.HValve 23", "FlowChart.HValve 24", "FlowChart.HValve 25", "FlowChart.HValve 26", "FlowChart.HValve 27", "FlowChart.HValve 28", "FlowChart.HValve 29", "FlowChart.HValve 30", "FlowChart.HValve 31", "FlowChart.HValve 32", "FlowChart.HValve 33", "FlowChart.HValve 34", "FlowChart.HValve 35", "FlowChart.HValve 36", "FlowChart.HValve 37", "FlowChart.HValve 38", "FlowChart.HValve 39", "FlowChart.HValve 40", "FlowChart.HValve 41", "FlowChart.HValve 42", "FlowChart.HValve 43", "FlowChart.HValve 44", "FlowChart.HValve 45", "FlowChart.HValve 46", "FlowChart.HValve 47", "FlowChart.HValve 48", "FlowChart.HValve 49", "FlowChart.HValve 50", "FlowChart.HValve 51", "FlowChart.HValve 52", "FlowChart.HValve 53", "FlowChart.HValve 54", "FlowChart.HValve 55", "FlowChart.HValve 56", "FlowChart.HValve 57", "FlowChart.HValve 58", "FlowChart.HValve 59", "FlowChart.HValve 60", "FlowChart.HValve 61", "FlowChart.HValve 62", "FlowChart.HValve 63", "FlowChart.HValve 64", "FlowChart.HValve 65", "FlowChart.HValve 66", "FlowChart.HValve 67", "FlowChart.HValve 68", "FlowChart.HValve 69", "FlowChart.HValve 70", "FlowChart.HValve 71", "FlowChart.HValve 72", "FlowChart.HValve 73", "FlowChart.HValve 74", "FlowChart.HValve 75", "FlowChart.HValve 76", "FlowChart.HValve 77", "FlowChart.HValve 78", "FlowChart.HValve 79", "FlowChart.HValve 80", "FlowChart.VValve 3", "FlowChart.VValve 4", "FlowChart.VValve 5", "FlowChart.VValve 6", "FlowChart.VValve 7", "FlowChart.VValve 8", "FlowChart.VValve 9", "FlowChart.VValve 10", "FlowChart.VValve 11", "FlowChart.VValve 12", "FlowChart.VValve 13", "FlowChart.VValve 14", "FlowChart.VValve 15", "FlowChart.VValve 16", "FlowChart.VValve 17", "FlowChart.VValve 18", "FlowChart.VValve 19", "FlowChart.VValve 20", "FlowChart.Bump 3", "FlowChart.Bump 4", "FlowChart.Bump 5", "FlowChart.Bump 6", "FlowChart.Bump 7", "FlowChart.Bump 8", "FlowChart.Bump 9", "FlowChart.Bump 10", "FlowChart.VFS 3", "FlowChart.VFS 4", "FlowChart.VFS 5", "FlowChart.VFS 6", "FlowChart.VFS 7", "FlowChart.VFS 8", "FlowChart.VFS 9", "FlowChart.VFS 10", "FlowChart.HFS 3", "FlowChart.HFS 4", "FlowChart.HFS 5", "FlowChart.HFS 6", "FlowChart.HFS 7", "FlowChart.HFS 8", "FlowChart.HFS 9", "FlowChart.HFS 10", "FlowChart.PRT 1", "FlowChart.PRT 2", "FlowChart.PRT 3", "FlowChart.PRT 4", "FlowChart.PRT 5", "FlowChart.PRT 6", "FlowChart.PRT 7", "FlowChart.PRT 8", "FlowChart.PRT 9", "FlowChart.PRT 10", "FlowChart.PRT 11", "FlowChart.PRT 12", "FlowChart.PRT 13", "FlowChart.PRT 14", "FlowChart.PRT 15", "FlowChart.PRT 16", "FlowChart.PRT 17", "FlowChart.PRT 18", "FlowChart.PRT 19", "FlowChart.PRT 20", "FlowChart.HVFS 1", "FlowChart.VVFS 1", "FlowChart.HVFS 2", "FlowChart.HVFS 3", "FlowChart.HVFS 4", "FlowChart.HVFS 5", "FlowChart.HVFS 6", "FlowChart.HVFS 7", "FlowChart.HVFS 8", "FlowChart.HVFS 9", "FlowChart.HVFS 10", "FlowChart.HVFS 11", "FlowChart.HVFS 12", "FlowChart.HVFS 13", "FlowChart.HVFS 14", "FlowChart.HVFS 15", "FlowChart.HVFS 16", "FlowChart.HVFS 17", "FlowChart.HVFS 18", "FlowChart.HVFS 19", "FlowChart.HVFS 20", "FlowChart.VVFS 2", "FlowChart.VVFS 3", "FlowChart.VVFS 4", "FlowChart.VVFS 5", "FlowChart.VVFS 6", "FlowChart.VVFS 7", "FlowChart.VVFS 8", "FlowChart.VVFS 9", "FlowChart.VVFS 10", "FlowChart.VVFS 11", "FlowChart.VVFS 12", "FlowChart.VVFS 13", "FlowChart.VVFS 14", "FlowChart.VVFS 15", "FlowChart.VVFS 16", "FlowChart.VVFS 17", "FlowChart.VVFS 18", "FlowChart.VVFS 19", "FlowChart.VVFS 20", "FlowChart.NHVFS 100", "FlowChart.NHFS 100", "FlowChart.NVFS 100", "FlowChart.NHVFS 101", "FlowChart.NVFS 101", "FlowChart.NHFS 101", "FlowChart.NHVFS 102", "FlowChart.NVFS 102", "FlowChart.NHFS 102", "FlowChart.NHVFS 103", "FlowChart.NVFS 103", "FlowChart.NHFS 103", "FlowChart.NHVFS 104", "FlowChart.NVFS 104", "FlowChart.NHFS 104", "FlowChart.NHVFS 105", "FlowChart.NVFS 105", "FlowChart.NHFS 105", "FlowChart.NHVFS 106", "FlowChart.NHFS 106", "FlowChart.NVFS 106", "FlowChart.NHVFS 107", "FlowChart.NVFS 107", "FlowChart.NHFS 107", "FlowChart.NHVFS 108", "FlowChart.NVFS 108", "FlowChart.NHFS 108", "FlowChart.NHVFS 109", "FlowChart.NVFS 109", "FlowChart.NHFS 109": Shortcut Menu Selection (User) {
        n15 = event-data() -> ("ItemTag"=w56:string, "Coords"=w49:T6, "CtlRef"=w47:refnum<vi>)  [unwired: 1 in]
        n16 = Bundle By Name(cluster=w55, "Init"=w49) -> (w52:T7)
        n17 = case shown="\"Bump\", \"Data\", \"HFS\", \"HVFS\", \"HValve\", \"LMG\", \"NHFS\", \"NHVFS\", \"NVFS\", \"PRT\", \"VFS\", \"VVFS\", \"VValve\"" w56 {
          selector: w56 -> [_ w70 _ _ _]
          tunnel: [_ w68 w79 _ _] -> w45
          tunnel: w52 -> [w66 w72 w80 w85 w90]
          tunnel: [w66 w72 w80 w85 w90] -> w54
          tunnel: w47 -> [_ _ w79 w81 w89]
          tunnel: w44 -> [w65 w67 w78 w84 w86]
          tunnel: [w65 w67 w78 w84 w86] -> w43
          frame Default {
          }
          frame "Bump", "Data", "HFS", "HVFS", "HValve", "LMG", "NHFS", "NHVFS", "NVFS", "PRT", "VFS", "VVFS", "VValve" {
            n18 = Unbundle By Name(w72) -> ("Type"=w71:map{string, map{string, refnum<vi>}})
            n19 = Look In Map(map=w71, key=w70) -> (value=w69:map{string, refnum<vi>})  [unwired: 1 in, 1 out]
            n20 = for {
              tunnel: w69 -> [w77] mode=indexing
              tunnel: [w75] -> w68 if=w73
              stop <- w73 stop-if-true
              n21 = Unbundle By Name(w77) -> ("Ref"=w76:refnum<vi>)
              n22 = property class="Ctl"(reference=w76) -> (reference out=w75:refnum<vi>, "Visible"=w74:bool)  [unwired: 1 in, 1 out]
              n23 = Not(x=w74) -> (.not. x?=w73:bool)
            }
          }
          frame "Move" {
          }
          frame "Edit" {
            n24 = Unbundle By Name(w84) -> ("UI"=w83:refnum<queue>)
            n25 = call "Queue In.vi"("Data"=w81, "Message"="Control Edit", "Queue In"=w83) -> ()  [unwired: 7 in, 2 out]
          }
          frame "Delete" {
            n26 = Unbundle By Name(w86) -> ("UI"=w88:refnum<queue>)
            n27 = call "Queue In.vi"("Data"=w89, "Message"="Control Hide", "Queue In"=w88) -> ()  [unwired: 7 in, 2 out]
          }
        }
        n28 = Not A Number/Path/Refnum?(number/path/refnum=w45) -> (NaN/Path/Refnum?=w46:bool)
        n29 = Not(x=w46) -> (.not. x?=w53:bool)
        n30 = Bundle By Name(cluster=w54, "ON?"=w53, "Object"=w45) -> (w51:T7)
        n31 = Unbundle By Name(w51) -> ("Init"=w42:T6, "Object"=w50:refnum<vi>, "ON?"=w48:bool)
        n32 = case shown="真" w48 {
          tunnel: w50 -> [_ w59]
          tunnel: w43 -> [_ w62]
          tunnel: w42 -> [_ w58]
          frame False {
          }
          frame True {
            n33 = Unbundle By Name(w62) -> ("Data"=w60:refnum<queue>)
            n34 = property class="Ctl"(reference=w59, "Position"=w58, "DisabledEnum"=T8."Disabled" ("禁用"), "Visible"=TRUE ("可见")) -> ("Label.Text"=w57:string)  [unwired: 1 in, 2 out]
            n35 = call "Queue In.vi"("Data"=w57, "Message"="Show", "Queue In"=w60) -> ()  [unwired: 7 in, 2 out]
          }
        }
      }
      event "FlowChart": Value Change {
        n36 = event-data() -> ("NewVal"=w96:T2, "OldVal"=w95:T2)  [unwired: 1 in]
        n37 = Unbundle By Name(w94) -> ("UI"=w93:refnum<queue>)
        n38 = call "FlowChart String Analize.vi"("Old Value"=w95, "New Value"=w96) -> ("Set"=w91:cluster{"Name":string, "Data":string})  [unwired: 7 in, 2 out]
        n39 = call "Queue In.vi"("Data"=w91, "Message"="Write Prepare", "Queue In"=w93) -> ()  [unwired: 7 in, 2 out]
      }
      event User Event {
        n40 = event-data() -> ("Type"=w98:map{string, map{string, refnum<vi>}})  [unwired: 1 in]
        n41 = Bundle By Name(cluster=w100, "Type"=w98) -> (w99:T7)
      }
      event "FlowChart": Mouse Move {
        n42 = event-data() -> ("Coords"=w101:T6)  [unwired: 1 in]
        n43 = Unbundle By Name(w103) -> ("ON?"=w104:bool)
        n44 = case shown="真" w104 {
          tunnel: w103 -> [w105 w115]
          tunnel: [w105 w115] -> w102
          tunnel: w101 -> [_ w114]
          frame False {
          }
          frame True {
            n45 = Unbundle By Name(w115) -> ("Object"=w112:refnum<vi>, "Init"=w111:T6)
            n46 = Subtract(x=w114, y=w111) -> (x-y=w113:T6)
            n47 = Add(x=w111, y=w113) -> (x+y=w109:T6)
            n48 = property class="Ctl"(reference=w112) -> (reference out=w110:refnum<vi>, "Bounds"=w108:T3)  [unwired: 1 in, 1 out]
            n49 = expression code="x/2"(w108) -> (w107:T3)
            n50 = Subtract(x=w109, y=w107) -> (x-y=w106:T3)
            n51 = property class="Ctl"(reference=w110, "Position"=w106) -> ()  [unwired: 1 in, 2 out]
          }
        }
      }
      event "FlowChart": Mouse Up {
        n52 = event-data() -> ()  [unwired: 1 in, 1 out]
        n53 = Unbundle By Name(w119) -> ("Object"=w117:refnum<vi>, "ON?"=w118:bool)
        n54 = case shown="真" w118 {
          tunnel: w117 -> [_ w127]
          tunnel: w116 -> [_ w125]
          frame False {
          }
          frame True {
            n55 = Unbundle By Name(w125) -> ("Data"=w124:refnum<queue>)
            n56 = property class="Ctl"(reference=w127, "DisabledEnum"=T8."Enabled" ("禁用")) -> ("Label.Text"=w123:string)  [unwired: 1 in, 2 out]
            n57 = call "Queue In.vi"("Data"=w123, "Message"="Position", "Queue In"=w124) -> ()  [unwired: 7 in, 2 out]
          }
        }
        n58 = Bundle By Name(cluster=w119, "ON?"=FALSE) -> (w121:T7)
      }
      event User Event {
        n59 = event-data() -> ("Message"=w131:string)  [unwired: 1 in]
        n60 = Equal?(x=w131, y="Exit") -> (x = y?=w129:bool)
      }
      event Panel Close? {
        n61 = event-data() -> ()  [unwired: 1 in, 1 out]
        n62 = Call Chain() -> (call chain=w137:string[])
        n63 = Array Size(array=w137) -> (size(s)=w136:i32)
        n64 = case shown="2, 默认" w136 {
          tunnel: w135 -> [w141 w144]
          tunnel: [w140 w143] -> w134
          tunnel: ["Panel Hidden" ("Message") "Exit Prepare" ("Message")] -> w133
          frame 2, Default {
            n65 = Unbundle By Name(w141) -> ("Message"=w140:refnum<queue>)
          }
          frame 1 {
            n66 = Unbundle By Name(w144) -> ("Message"=w143:refnum<queue>)
          }
        }
        n67 = call "Queue In.vi"("Message"=w133, "Queue In"=w134) -> ()  [unwired: 8 in, 2 out]
        n68 = event-data("Discard?"=TRUE ("放弃？")) -> ()  [unwired: 1 in, 1 out]
      }
      event Panel Resize {
        n69 = event-data() -> ()  [unwired: 1 in, 1 out]
        n70 = Unbundle By Name(w147) -> ("UI"=w146:refnum<queue>)
        n71 = call "Queue In.vi"("Message"="Panel Change", "Queue In"=w146) -> ()  [unwired: 8 in, 2 out]
      }
      event "Panel Show": Value Change {
        n72 = event-data() -> ("CtlRef"=w150:refnum<vi>)  [unwired: 1 in]
        n73 = Unbundle By Name(w152) -> ("Message"=w151:refnum<queue>)
        n74 = property class="Bool"(reference=w150) -> ("Label.Text"=w149:string)  [unwired: 1 in, 2 out]
        n75 = call "Queue In.vi"("Message"=w149, "Queue In"=w151) -> ()  [unwired: 8 in, 2 out]
      }
      event "Picture Add", "Picture Delete", "Vertical scroll bar", "Horizontal scroll bar", "FlowChartEdit", "Load Picture", "WorkMode Edit", "ShowLable", "LogRead": Value Change {
        n76 = event-data() -> ("CtlRef"=w157:refnum<vi>)  [unwired: 1 in]
        n77 = Unbundle By Name(w156) -> ("UI"=w155:refnum<queue>)
        n78 = property class="Bool"(reference=w157) -> ("Label.Text"=w154:string)  [unwired: 1 in, 2 out]
        n79 = call "Queue In.vi"("Message"=w154, "Queue In"=w155) -> ()  [unwired: 8 in, 2 out]
      }
      event "Chart Select": Value Change {
        n80 = event-data() -> ("CtlRef"=w162:refnum<vi>)  [unwired: 1 in]
        n81 = property class="Ring (严格)"(reference=w162) -> ("Label.Text"=w159:string)  [unwired: 1 in, 2 out]
        n82 = Unbundle By Name(w161) -> ("UI"=w160:refnum<queue>)
        n83 = call "Queue In.vi"("Message"=w159, "Queue In"=w160) -> ()  [unwired: 8 in, 2 out]
      }
    }
  }
  n84 = while {
    tunnel: w15 -> [w175]
    tunnel: [w172] -> w17
    tunnel: [w171] -> w16
    shift-right: [w167] -> _
    shift-left: T5 {"Queue"={"UI"=refnum, "Message"=refnum, "Data"=refnum, "Caller"=refnum, "Name"="000 Common", "Data Path"=path "", "Class Path"=path "", "SubPanel"=refnum, "Project Name"="", "MNT"="", "Title"="", "Data Source"=refnum, "Queue List"={}, "VI"=refnum, "UE"=refnum}, "Delay"={"Count Time(ms)"=250, "Delay Time(ms)"=250, "Next"="Receive Data,Delay"}, "Panel"=refnum, "Property"={}, "File"=path "FlowChart.csv", "CPicture"="", "Mode"={"Mode"="", "Data"="-1"}} -> [w166]
    tunnel: w3 -> [w164]
    stop <- w179 stop-if-true
    n85 = call "Queue Out.vi"("Queue In"=w175) -> ("error out"=w178:errorcluster, "Data"=w176:variant, "Message"=w177:string, "Queue Out"=w174:refnum<queue>, "Queue NUmber"=w165:i32)  [unwired: 6 in]
    n86 = case shown="\"Log\"" w177 {
      selector: w177 -> [_ _ w228 _ _ _ w382 _ _ _ _ w524 _ w535 _ _]
      tunnel: w174 -> [w184 w197 w234 w272 w308 w377 w386 w410 w437 w468 w522 w531 w534 w540 w555 w574]
      tunnel: w178 -> [w183 w196 w233 w271 w307 w376 w385 w409 w436 w467 w521 w530 w533 w539 w553 w575]
      tunnel: [w184 w197 w234 w272 w308 w377 w386 w410 w437 w468 w522 w531 w534 w540 w554 w574] -> w173
      tunnel: [w183 w196 w233 w271 w307 w376 w385 w409 w436 w467 w521 w530 w533 w539 w552 w575] -> w170
      tunnel: [w182 "Delay" ("Next") "Save Config" ("Next") "Save Config,Load Picture" ("Next") "Refresh Control" ("Next") _ _ _ _ _ _ w525 _ _ "Quit" _] -> w169
      tunnel: [_ _ _ _ _ _ _ _ _ _ _ _ _ _ _ TRUE] -> w179
      tunnel: [w181 _ _ _ _ _ _ _ _ _ _ _ _ _ _ _] -> w168
      tunnel: w176 -> [_ _ w232 w270 w303 w374 w381 _ _ _ w519 _ _ w536 _ _]
      tunnel: [w180 w193 w230 w264 w305 w364 w384 w388 w434 w465 w520 w523 w532 w537 w550 w572] -> w167
      tunnel: w166 -> [w180 w195 w226 w268 w284 w375 w384 w388 w434 w449 w520 w523 w532 w538 w550 w572]
      tunnel: w165 -> [_ _ _ _ _ _ _ _ _ _ _ _ _ _ _ _]
      tunnel: w164 -> [_ w194 _ _ _ _ _ _ _ _ _ _ _ _ _ _]
      frame Default {
        w181 = variant  # Data
        w182 = ""  # Message
      }
      frame "Init" {
        n87 = Bundle By Name(cluster=w195, "Queue"=w194) -> (w190:T5)
        n88 = Unbundle By Name(w190) -> ("Queue.VI"=w189:refnum<vi>)
        n89 = property class="VI"(reference=w189) -> ("Panel"=w188:refnum<vi>)  [unwired: 1 in, 2 out]
        n90 = property class="Pnl"(reference=w188, "DeferPanUpdts"=TRUE ("延迟前面板更新")) -> (reference out=w186:refnum<vi>)  [unwired: 1 in, 1 out]
        n91 = flat-sequence {
          tunnel: w190 -> [w203]
          tunnel: [w201] -> w191
          tunnel: w186 -> [w200]
          tunnel: [w200] -> w185
          tunnel: [w225] -> w193
          tunnel: w191 -> [w225]
          tunnel: w185 -> [w223]
          frame #0 {
            n92 = control-ref of="FlowChart"() -> (w206:refnum<vi>)
            n93 = property class="Clust (严格)"(reference=w206) -> ("Controls[]"=w207:refnum<vi>[])  [unwired: 1 in, 2 out]
            n94 = Unbundle By Name(w203) -> ("Property"=w205:T13)
            n95 = for {
              tunnel: w207 -> [w214] mode=indexing
              shift-right: [w211] -> w204
              shift-left: w205 -> [w213]
              tunnel: T11 {"Left"=0, "Top"=0} ("位置") -> [w209]
              tunnel: FALSE -> [w208]
              n96 = property class="Ctl"(reference=w214, "Position"=w209, "Visible"=w208, "Label.Visible"=w208) -> (reference out=w212:refnum<vi>, "Label.Text"=w210:string)  [unwired: 1 in, 1 out]
              n97 = in-place {
                in-place-border: w212 -> [w220]
                in-place-border: w210 -> [w219]
                n98 = in-place-map #1(w213, w210) -> (w222:T14)  [unwired: 1 in, 1 out]
                n99 = call <vilib>:"Delimited String to 1D String Array.vi"("delimiter"=" ", "delimited string"=w219) -> ("string array"=w217:string[])  [unwired: 9 in]
                n100 = Index Array(array=w217) -> (element=w216:string)  [unwired: 1 in]
                n101 = Bundle By Name(cluster=w222, "Ref"=w220, "Control"=w219, "Type"=w216) -> (w221:T14)
                n102 = in-place-map #1(w221, LVMapReplaceAction."Add or Modify Entry" ("操作")) -> (w211:T13)  [unwired: 2 out]
              }
            }
            n103 = control-ref of="Panel"() -> (w202:refnum<vi>)
            n104 = Bundle By Name(cluster=w203, "Property"=w204, "Panel"=w202) -> (w201:T5)
          }
          frame #1 {
            n105 = property class="Pnl"(reference=w223, "DeferPanUpdts"=FALSE ("延迟前面板更新")) -> ()  [unwired: 1 in, 2 out]
          }
        }
      }
      frame "Hide", "Position", "Show" {
        n106 = Variant To Data(type="", Variant=w232) -> (data=w229:string)  [unwired: 1 in, 1 out]
        n107 = in-place {
          in-place-border: w229 -> [w236]
          in-place-border: w228 -> [w235]
          n108 = in-place-cluster #2(w226) -> ("Property"=w238:T13)
          n109 = in-place {
            in-place-border: w235 -> [w241]
            n110 = in-place-map #3(w238, w236) -> (w240:T14)  [unwired: 1 in, 1 out]
            n111 = case shown="\"Hide\"" w241 {
              tunnel: w240 -> [w242 w245 w250 w255 w258]
              tunnel: [w242 w244 w248 w253 w257] -> w239
              frame Default {
              }
              frame "Hide" {
                n112 = Bundle By Name(cluster=w245, "Show"=FALSE) -> (w244:T14)
              }
              frame "Position" {
                n113 = Unbundle By Name(w250) -> ("Ref"=w249:refnum<vi>)
                n114 = property class="Ctl"(reference=w249) -> ("Left"=w247:i32, "Top"=w246:i32)  [unwired: 1 in, 2 out]
                n115 = Bundle By Name(cluster=w250, "Left"=w247, "Top"=w246) -> (w248:T14)
              }
              frame "ID" {
                n116 = Unbundle By Name(w255) -> ("Ref"=w254:refnum<vi>)
                n117 = property class="Ctl"(reference=w254) -> ("Desc"=w252:string, "TipStrip"=w251:string)  [unwired: 1 in, 2 out]
                n118 = Bundle By Name(cluster=w255, "ID"=w252, "Name"=w251) -> (w253:T14)
              }
              frame "Show" {
                n119 = Bundle By Name(cluster=w258, "Show"=TRUE) -> (w257:T14)
              }
            }
            n120 = in-place-map #3(w239) -> (w237:T13)  [unwired: 1 in, 2 out]
          }
          n121 = in-place-cluster #2("Property"=w237) -> (w230:T5)
        }
      }
      frame "ID Change" {
        n122 = Variant To Data(type="", Variant=w270) -> (data=w263:string)  [unwired: 1 in, 1 out]
        n123 = Unbundle By Name(w268) -> ("Property"=w267:T13)
        n124 = Look In Map(map=w267, key=w263) -> (value=w266:T14)  [unwired: 1 in, 1 out]
        n125 = Unbundle By Name(w266) -> ("Ref"=w265:refnum<vi>)
        n126 = property class="Ctl"(reference=w265) -> ("Label.Text"=w262:string, "Desc"=w261:string, "TipStrip"=w260:string)  [unwired: 1 in, 2 out]
        n127 = in-place {
          in-place-border: w262 -> [w275]
          in-place-border: w261 -> [w274]
          in-place-border: w260 -> [w273]
          n128 = in-place-cluster #4(w268) -> ("Property"=w277:T13)
          n129 = in-place {
            in-place-border: w274 -> [w280]
            in-place-border: w273 -> [w279]
            n130 = in-place-map #5(w277, w275) -> (w281:T14)  [unwired: 1 in, 1 out]
            n131 = Bundle By Name(cluster=w281, "ID"=w280, "Name"=w279) -> (w278:T14)
            n132 = in-place-map #5(w278) -> (w276:T13)  [unwired: 1 in, 2 out]
          }
          n133 = in-place-cluster #4("Property"=w276) -> (w264:T5)
        }
      }
      frame "Load Config" {
        n134 = in-place {
          in-place-border: w303 -> [w362]
          n135 = in-place-cluster #6(w284) -> ("CPicture"=w361:string)
          n136 = Variant To Data(type=w361, Variant=w362) -> (data=w360:string)  [unwired: 1 in, 1 out]
          n137 = in-place-cluster #6("CPicture"=w360) -> (w304:T5)
        }
        n138 = Unbundle By Name(w284) -> ("Queue.Data Path"=w288:path)
        n139 = Build Path(base path=w288, name or relative path=path "Config.ini" ("名称或相对路径")) -> (appended path=w289:path)
        n140 = Unbundle By Name(w304) -> ("Queue.Data Path"=w302:path, "CPicture"=w299:string)
        n141 = call <vilib>:"Open Config Data.vi"("configuration file path"=w289) -> ("error out"=w292:errorcluster, "refnum"=w293:T15)  [unwired: 8 in, 1 out]
        n142 = Build Path(base path=w302, name or relative path=w299) -> (appended path=w301:path)
        n143 = call-poly <vilib>:"Read Key.vi"("section"="FlowChart", "error in (no error)"=w292, "key"="Mode", "refnum"=w293) -> ("error out"=w290:errorcluster, "value"=w282:string, "refnum out"=w291:T15)  [unwired: 4 in, 1 out]
        n144 = Format Into String(format string="%s.csv" ("格式字符串"), w299) -> (resulting string=w298:string)  [unwired: 2 in, 1 out]
        n145 = Build Path(base path=w301, name or relative path=w298) -> (appended path=w297:path)
        n146 = call <vilib>:"Close Config Data.vi"("error in (no error)"=w290, "refnum"=w291) -> ()  [unwired: 8 in, 2 out]
        n147 = Bundle By Name(cluster=w304, "Mode.Mode"=w282) -> (w283:T5)
        n148 = call <vilib>:"Check if File or Folder Exists.vi"("path"=w297) -> ("error out"=w294:errorcluster, "file or folder exists?"=w296:bool, "dup path"=w295:path)  [unwired: 8 in]
        n149 = case shown="真" w296 {
          tunnel: [w309 w317] -> w305
          tunnel: w283 -> [w310 w323]
          tunnel: w295 -> [_ w322]
          tunnel: w294 -> [_ w321]
          frame False {
            n150 = in-place {
              n151 = in-place-cluster #7(w310) -> ("Property"=w312:T13)
              n152 = in-place {
                n153 = in-place-map #8(w312) -> (w315:T14)  [unwired: 2 in, 1 out]
                n154 = Bundle By Name(cluster=w315, "Show"=FALSE) -> (w314:T14)
                n155 = in-place-map #8(w314) -> (w311:T13)  [unwired: 1 in, 2 out]
              }
              n156 = in-place-cluster #7("Property"=w311) -> (w309:T5)
            }
          }
          frame True {
            n157 = call-poly <vilib>:"Read Delimited Spreadsheet.vi"("file path (dialog if empty)"=w322, "error in (no error)"=w321, "delimiter (\\t)"="," ("delimiter (\\t)")) -> ("all rows"=w330:string[][])  [unwired: 7 in, 5 out]
            n158 = Delete From Array(array=w330, length=1 ("长度"), index (row)=0 ("索引 (行)")) -> (array with subset deleted=w327:string[][])  [unwired: 1 in, 1 out]
            n159 = for {
              tunnel: w327 -> [w332] mode=indexing
              shift-right: [w333] -> w317
              shift-left: w323 -> [w334]
              n160 = in-place {
                in-place-border: w332 -> [w349]
                n161 = in-place-cluster #9(w334) -> ("Property"=w350:T13)
                n162 = Index Array(array=w349) -> (element #1=w348:string, element #2=w335:string, element #3=w347:string, element #4=w346:string, element #5=w345:string, element #6=w341:string, element #7=w337:string)  [unwired: 7 in]
                n163 = Fract/Exp String To Number(string=w341, default (0 dbl)=0 ("Top")) -> (number=w339:i32)  [unwired: 2 in, 1 out]
                n164 = Fract/Exp String To Number(string=w337, default (0 dbl)=0 ("Top")) -> (number=w336:i32)  [unwired: 2 in, 1 out]
                n165 = Equal?(x=w345, y="1") -> (x = y?=w343:bool)
                n166 = in-place {
                  in-place-border: w348 -> [w358]
                  in-place-border: w335 -> [w357]
                  in-place-border: w347 -> [w356]
                  in-place-border: w346 -> [w355]
                  in-place-border: w343 -> [w354]
                  in-place-border: w339 -> [w352]
                  in-place-border: w336 -> [w351]
                  n167 = in-place-map #10(w350, w335) -> (w359:T14)  [unwired: 1 in, 1 out]
                  n168 = Bundle By Name(cluster=w359, "Type"=w358, "Control"=w357, "Name"=w356, "ID"=w355, "Show"=w354, "Top"=w352, "Left"=w351) -> (w353:T14)
                  n169 = in-place-map #10(w353) -> (w342:T13)  [unwired: 1 in, 2 out]
                }
                n170 = in-place-cluster #9("Property"=w342) -> (w333:T5)
              }
            }
            n171 = Unbundle By Name(w317) -> ("Queue.UI"=w326:refnum<queue>, "Property"=w324:T13)
            n172 = Unbundle By Name(w317) -> ("Mode.Mode"=w316:string)
            n173 = call "Queue In.vi"("Data"=w324, "Message"="Control Refer", "Queue In"=w326) -> ("error out"=w319:errorcluster, "Queue Out"=w320:refnum<queue>)  [unwired: 7 in]
            n174 = call "Queue In.vi"("error in (no error)"=w319, "Data"=w316, "Message"="WorkMode", "Queue In"=w320) -> ()  [unwired: 6 in, 2 out]
          }
        }
      }
      frame "WorkMode" {
        n175 = in-place {
          in-place-border: w374 -> [w380]
          in-place-border: [w378] -> w363
          n176 = in-place-cluster #11(w375) -> ("Mode.Mode"=w379:string)
          n177 = Variant To Data(type=w379, Variant=w380) -> (data=w378:string)  [unwired: 1 in, 1 out]
          n178 = in-place-cluster #11("Mode.Mode"=w378) -> (w364:T5)
        }
        n179 = Unbundle By Name(w364) -> ("Queue.Data Path"=w368:path)
        n180 = Build Path(base path=w368, name or relative path=path "Config.ini" ("名称或相对路径")) -> (appended path=w369:path)
        n181 = call <vilib>:"Open Config Data.vi"("configuration file path"=w369) -> ("error out"=w372:errorcluster, "refnum"=w373:T15)  [unwired: 8 in, 1 out]
        n182 = call-poly <vilib>:"Write Key.vi"("section"="FlowChart", "error in (no error)"=w372, "value"=w363, "key"="Mode", "refnum"=w373) -> ("error out"=w370:errorcluster, "refnum out"=w371:T15)  [unwired: 4 in, 1 out]
        n183 = call <vilib>:"Close Config Data.vi"("error in (no error)"=w370, "refnum"=w371) -> ()  [unwired: 8 in, 2 out]
      }
      frame "Load Picture" {
        n184 = Unbundle By Name(w384) -> ("Queue.UI"=w383:refnum<queue>)
        n185 = call "Queue In.vi"("Data"=w381, "Message"=w382, "Queue In"=w383) -> ()  [unwired: 7 in, 2 out]
      }
      frame "Save Config" {
        n186 = Unbundle By Name(w388) -> ("Property"=w408:T13)
        n187 = for {
          tunnel: w408 -> [w426] mode=indexing
          tunnel: [w411] -> w405 mode=indexing
          n188 = Unbundle By Name(w426) -> ("Data.Type"=w418:string, "Data.Control"=w417:string, "Data.Name"=w416:string, "Data.ID"=w415:string, "Data.Show"=w425:bool, "Data.Top"=w421:i32, "Data.Left"=w419:i32)
          n189 = Select(t="1", s=w425, f="0") -> (s? t:f=w414:string)
          n190 = Format Into String(format string="%d" ("格式字符串"), w421) -> (resulting string=w413:string)  [unwired: 2 in, 1 out]
          n191 = Format Into String(format string="%d" ("格式字符串"), w419) -> (resulting string=w412:string)  [unwired: 2 in, 1 out]
          n192 = Build Array(w418, w417, w416, w415, w414, w413, w412) -> (w411:string[])
        }
        n193 = Unbundle By Name(w388) -> ("Queue.Data Path"=w402:path, "CPicture"=w399:string)
        n194 = Build Array (concatenate)(string[] ["Type", "Control", "Name", "ID", "Show", "Top", "Left"], w405) -> (w404:string[][])
        n195 = Build Path(base path=w402, name or relative path=w399) -> (appended path=w401:path)
        n196 = Format Into String(format string="%s.csv" ("格式字符串"), w399) -> (resulting string=w398:string)  [unwired: 2 in, 1 out]
        n197 = Build Path(base path=w401, name or relative path=w398) -> (appended path=w403:path)
        n198 = call-poly <vilib>:"Write Delimited Spreadsheet.vi"("file path (dialog if empty)"=w403, "2D data"=w404, "delimiter (\\t)"="," ("delimiter (\\t)")) -> ()  [unwired: 11 in, 2 out]
        n199 = Unbundle By Name(w388) -> ("Queue.Data Path"=w393:path)
        n200 = Unbundle By Name(w388) -> ("CPicture"=w387:string)
        n201 = Build Path(base path=w393, name or relative path=path "Config.ini" ("名称或相对路径")) -> (appended path=w392:path)
        n202 = call <vilib>:"Open Config Data.vi"("configuration file path"=w392) -> ("error out"=w397:errorcluster, "refnum"=w391:T15)  [unwired: 8 in, 1 out]
        n203 = call-poly <vilib>:"Write Key.vi"("section"="FlowChart", "error in (no error)"=w397, "value"=w387, "key"="Current_Picture", "refnum"=w391) -> ("error out"=w396:errorcluster, "refnum out"=w390:T15)  [unwired: 4 in, 1 out]
        n204 = call <vilib>:"Close Config Data.vi"("error in (no error)"=w396, "refnum"=w390) -> ()  [unwired: 8 in, 2 out]
      }
      frame "Refresh Control" {
        n205 = Unbundle By Name(w434) -> ("Property"=w435:T13, "Panel"=w433:refnum<vi>)
        n206 = property class="Pane"(reference=w433) -> ("OwningVI"=w432:refnum<vi>)  [unwired: 1 in, 2 out]
        n207 = property class="VI"(reference=w432) -> ("Panel"=w431:refnum<vi>)  [unwired: 1 in, 2 out]
        n208 = property class="Pnl"(reference=w431, "DeferPanUpdts"=TRUE ("延迟前面板更新")) -> (reference out=w429:refnum<vi>)  [unwired: 1 in, 1 out]
        n209 = for {
          tunnel: w435 -> [w448] mode=indexing
          shift-right: [w440] -> _
          shift-left: w434 -> [w440]
          shift-right: [w438] -> w427
          shift-left: w429 -> [w438]
          n210 = Unbundle By Name(w448) -> ("Data.Ref"=w442:refnum<vi>, "Data.Name"=w441:string, "Data.Name"=w443:string, "Data.ID"=w447:string, "Data.Left"=w446:i32, "Data.Top"=w445:i32, "Data.Show"=w444:bool)
          n211 = Bundle("Left"=w446, "Top"=w445) -> (w439:cluster{"Left":i32, "Top":i32})  [unwired: 1 in]
          n212 = property class="Ctl"(reference=w442, "Caption.Text"=w441, "TipStrip"=w443, "Desc"=w447, "Position"=w439, "Visible"=w444) -> ()  [unwired: 1 in, 2 out]
        }
        n213 = property class="Pnl"(reference=w427, "DeferPanUpdts"=FALSE ("延迟前面板更新")) -> ()  [unwired: 1 in, 2 out]
      }
      frame "Receive Data" {
        n214 = Unbundle By Name(w449) -> ("Queue.Project Name"=w466:string, "Property"=w464:T13, "Mode.Mode"=w461:string, "Mode.Data"=w457:string)
        n215 = Unbundle By Name(w449) -> ("Queue.VI"=w453:refnum<vi>)
        n216 = property class="VI"(reference=w453) -> ("Panel"=w455:refnum<vi>)  [unwired: 1 in, 2 out]
        n217 = call "Data Global.vi"("Name"=w466) -> ("Data Out"=w463:map{string, T16})  [unwired: 7 in, 3 out]
        n218 = property class="Pnl"(reference=w455, "DeferPanUpdts"=TRUE ("延迟前面板更新")) -> (reference out=w452:refnum<vi>)  [unwired: 1 in, 1 out]
        n219 = Look In Map(map=w463, key=w461) -> (value=w462:T16)  [unwired: 1 in, 1 out]
        n220 = Unbundle By Name(w462) -> ("Data"=w458:string)
        n221 = Not Equal?(x=w458, y=w457) -> (x != y?=w460:bool)
        n222 = case shown="真" w460 {
          tunnel: w449 -> [w469 w473]
          tunnel: [w469 w473] -> w459
          tunnel: w458 -> [_ w470]
          frame False {
          }
          frame True {
            n223 = Unbundle By Name(w473) -> ("Queue.UI"=w472:refnum<queue>)
            n224 = call "Queue In.vi"("Data"=w470, "Message"="Mode Change", "Queue In"=w472) -> ()  [unwired: 7 in, 2 out]
          }
        }
        n225 = Bundle By Name(cluster=w459, "Mode.Data"=w458) -> (w456:T5)
        n226 = for {
          tunnel: w464 -> [w479] mode=indexing
          shift-right: [w478] -> w465
          shift-left: w456 -> [w478]
          tunnel: w463 -> [w477]
          shift-right: [w474] -> w450
          shift-left: w452 -> [w474]
          n227 = Unbundle By Name(w479) -> ("Data.Ref"=w476:refnum<vi>, "Data.Show"=w475:bool)
          n228 = case shown="真" w475 {
            tunnel: w477 -> [_ w481]
            tunnel: w476 -> [_ w480]
            frame False {
            }
            frame True {
              n229 = property class="Ctl"(reference=w480) -> (reference out=w484:refnum<vi>, "Desc"=w482:string, "ClassName"=w483:string)  [unwired: 1 in, 1 out]
              n230 = case shown="默认" w482 {
                selector: w482 -> [w487 _]
                tunnel: w484 -> [w490 _]
                tunnel: w483 -> [w489 _]
                tunnel: w481 -> [w486 _]
                frame Default {
                  n231 = Look In Map(map=w486, key=w487) -> (value=w488:T16)  [unwired: 1 in, 1 out]
                  n232 = Unbundle By Name(w488) -> ("Data"=w491:string, "Unit"=w492:string)
                  n233 = case shown="\"Boolean\"" w489 {
                    tunnel: w490 -> [_ w495 w503]
                    tunnel: w491 -> [_ w494 w502]
                    tunnel: w492 -> [_ _ w497]
                    tunnel: "Decimal" -> [_ _ w500]
                    frame "eee", Default {
                    }
                    frame "Boolean" {
                      n234 = call "000_Bool True.vi"("Bool String"=w494) -> ("True"=w493:bool)  [unwired: 8 in, 2 out]
                      n235 = property class="Ctl"(reference=w495, "Value"=w493) -> ()  [unwired: 1 in, 2 out]
                    }
                    frame "String" {
                      n236 = Fract/Exp String To Number(string=w502) -> (number=w501:dbl)  [unwired: 3 in, 1 out]
                      n237 = Number To Fractional String(number=w501, precision (6)=w500) -> (F-format string=w498:string)  [unwired: 2 in]
                      n238 = Concatenate Strings(w498, " " ("字符串"), w497) -> (w496:string)
                      n239 = property class="Ctl"(reference=w503, "Value"=w496) -> ()  [unwired: 1 in, 2 out]
                    }
                  }
                }
                frame "" {
                }
              }
            }
          }
        }
        n240 = property class="Pnl"(reference=w450, "DeferPanUpdts"=FALSE ("延迟前面板更新")) -> ()  [unwired: 1 in, 2 out]
      }
      frame "Log" {
        n241 = Unbundle By Name(w520) -> ("Queue.Data Path"=w512:path)
        n242 = Variant To Data(type="", Variant=w519) -> (data=w516:string)  [unwired: 1 in, 1 out]
        n243 = Format Date/Time String(time format string (%c)="%Y/%m/%d_%H:%M:%S" ("时间格式字符串(%c)")) -> (date/time string=w515:string)  [unwired: 2 in]
        n244 = Build Path(base path=w512, name or relative path=path "Log" ("名称或相对路径")) -> (appended path=w511:path)
        n245 = Format Into String(format string="%s %s" ("格式字符串"), w516, w515) -> (resulting string=w513:string)  [unwired: 2 in, 1 out]
        n246 = Format Date/Time String(time format string (%c)="%Y%m%d.txt" ("时间格式字符串(%c)")) -> (date/time string=w505:string)  [unwired: 2 in]
        n247 = call "Directory Create.vi"("folder path In"=w511) -> ("folder path out"=w510:path)  [unwired: 9 in, 1 out]
        n248 = Build Path(base path=w510, name or relative path=w505) -> (appended path=w509:path)
        n249 = Concatenate Strings(w513, "\r") -> (w507:string)
        n250 = call "000 Write TXT.vi"("txt"=w507, "Path"=w509) -> ()  [unwired: 9 in, 1 out]
      }
      frame "Delay" {
        n251 = Unbundle By Name(w523) -> ("Delay.Next"=w529:string, "Delay.Count Time(ms)"=w526:u32, "Delay.Delay Time(ms)"=w527:u32)
        n252 = call "Delay Judge.vi"("Delay Time(ms)"=w527, "Count Time(ms)"=w526) -> ("Time Out?"=w528:bool)  [unwired: 5 in, 4 out]
        n253 = Select(t=w529, s=w528, f=w524) -> (s? t:f=w525:string)
      }
      frame "====System====" {
      }
      frame "Refresh Class Ref" {
        n254 = case shown="\"Refresh Class Ref\"" w535 {
          tunnel: w538 -> [w541 w544]
          tunnel: [w541 w543] -> w537
          tunnel: w536 -> [_ w542]
          frame "eee", Default {
          }
          frame "Refresh Class Ref" {
            n255 = in-place {
              in-place-border: w542 -> [w547]
              n256 = in-place-cluster #12(w544) -> ("Queue"=w546:T1)
              n257 = Variant To Data(type=w546, Variant=w547) -> (data=w545:T1)  [unwired: 1 in, 1 out]
              n258 = in-place-cluster #12("Queue"=w545) -> (w543:T5)
            }
          }
        }
      }
      frame "Exit" {
        n259 = flat-sequence {
          tunnel: w550 -> [w562]
          tunnel: [w562] -> w551
          tunnel: w550 -> [w558]
          tunnel: [w557] -> w548
          tunnel: w551 -> [w565]
          tunnel: [w563] -> w549
          tunnel: w548 -> [w563]
          tunnel: w549 -> [w570]
          frame #0 {
            n260 = Unbundle By Name(w558) -> ("Queue.VI"=w561:refnum<vi>)
            n261 = property class="VI"(reference=w561) -> ("Panel"=w560:refnum<vi>)  [unwired: 1 in, 2 out]
            n262 = property class="Pnl"(reference=w560, "DeferPanUpdts"=TRUE ("延迟前面板更新")) -> (reference out=w557:refnum<vi>)  [unwired: 1 in, 1 out]
          }
          frame #1 {
            n263 = Unbundle By Name(w565) -> ("Property"=w564:T13)
            n264 = for {
              tunnel: w564 -> [w569] mode=indexing
              w567 = TRUE ("标签.可见")
              n265 = Unbundle By Name(w569) -> ("Data.Ref"=w568:refnum<vi>)
              n266 = property class="Ctl"(reference=w568, "Label.Visible"=w567, "Visible"=w567, "Caption.Visible"=FALSE ("标题.可见")) -> ()  [unwired: 1 in, 2 out]
            }
          }
          frame #2 {
            n267 = property class="Pnl"(reference=w570, "DeferPanUpdts"=FALSE ("延迟前面板更新")) -> ()  [unwired: 1 in, 2 out]
          }
        }
        n268 = call "Queue Clear.vi"("error in (no error)"=w553, "Queue In"=w555) -> ("error out"=w552:errorcluster, "Queue Out"=w554:refnum<queue>)  [unwired: 8 in]
      }
      frame "Quit" {
      }
    }
    n269 = call "Queue In.vi"("error in (no error)"=w170, "Data"=w168, "Message"=w169, "Queue In"=w173) -> ("error out"=w171:errorcluster, "Queue Out"=w172:refnum<queue>)  [unwired: 6 in]
  }
  n270 = while {
    tunnel: w23 -> [w586]
    tunnel: [w583] -> w25
    tunnel: [w582] -> w24
    shift-right: [w578] -> _
    shift-left: w5 -> [w577]
    tunnel: w3 -> [w576]
    stop <- w590 stop-if-true
    n271 = call "Queue Out.vi"("Queue In"=w586) -> ("error out"=w589:errorcluster, "Data"=w587:variant, "Message"=w588:string, "Queue Out"=w585:refnum<queue>)  [unwired: 6 in, 1 out]
    n272 = case shown="\"Picture Add\"" w588 {
      selector: w588 -> [_ _ _ _ _ _ _ _ _ _ _ _ _ _ _ _ _ _ _ _ w979 w994 _]
      tunnel: w585 -> [w595 w604 w618 w646 w687 w699 w710 w724 w747 w787 w799 w807 w824 w878 w902 w914 w933 w966 w975 w978 w984 w1001 w1007]
      tunnel: w589 -> [w594 w603 w617 w645 w686 w698 w709 w723 w746 w786 w798 w806 w823 w877 w901 w913 w932 w965 w974 w977 w983 w999 w1008]
      tunnel: [w595 w604 w618 w646 w687 w699 w710 w724 w747 w787 w799 w807 w824 w878 w902 w914 w933 w966 w975 w978 w984 w1000 w1007] -> w584
      tunnel: [w594 w603 w617 w645 w686 w698 w709 w723 w746 w786 w798 w806 w823 w877 w901 w913 w932 w965 w974 w977 w983 w998 w1008] -> w581
      tunnel: [w593 "Load Picture" ("Message") "Panel Change" ("Message") w627 _ _ _ _ _ _ _ _ _ w870 _ _ _ _ _ _ _ "Quit" _] -> w580
      tunnel: [_ _ _ _ _ _ _ _ _ _ _ _ _ _ _ _ _ _ _ _ _ _ TRUE] -> w590
      tunnel: [w592 _ _ _ _ _ _ _ _ _ _ _ _ _ _ _ _ _ _ _ _ _ _] -> w579
      tunnel: w587 -> [_ _ _ _ w684 w696 _ _ w745 _ _ _ _ _ w896 _ w930 w963 _ _ w980 _ _]
      tunnel: [w591 w601 w606 w635 w683 w692 w706 w721 w743 w785 w797 w805 w821 w871 w897 w911 w926 w964 w973 w976 w981 w993 w1005] -> w578
      tunnel: w577 -> [w591 w602 w616 w644 w685 w697 w703 w721 w743 w785 w797 w805 w822 w872 w897 w912 w931 w964 w973 w976 w982 w993 w1005]
      tunnel: w576 -> [_ w600 _ _ _ _ _ _ _ _ _ _ _ _ _ _ _ _ _ _ _ _ _]
      frame Default {
        w592 = variant  # Data
        w593 = ""  # Message
      }
      frame "Init" {
        n273 = control-ref of="Chart Select"() -> (w596:refnum<vi>)
        n274 = control-ref of="Panel"() -> (w598:refnum<vi>)
        n275 = control-ref of="Picture"() -> (w597:refnum<vi>)
        n276 = Bundle By Name(cluster=w602, "Queue"=w600, "Panel"=w598, "Picture"=w597, "Chart Select"=w596) -> (w601:T4)
      }
      frame "Horizontal scroll bar", "Vertical scroll bar" {
        w611 = T17."Always Off" ("垂直滚动条可见")
        w612 = T17."Always On" ("垂直滚动条可见")
        n277 = Unbundle By Name(w616) -> ("Panel"=w615:refnum<vi>)
        n278 = Select(t=w612, s="Horizontal scroll bar", f=w611) -> (s? t:f=w610:T17)
        n279 = Select(t=w612, s="Vertical scroll bar", f=w611) -> (s? t:f=w613:T17)
        n280 = property class="Pane"(reference=w615, "VertScrollbarVisibility"=w613) -> (reference out=w614:refnum<vi>)  [unwired: 1 in, 1 out]
        n281 = property class="Pane"(reference=w614, "HorizScrollbarVisibility"=w610) -> ()  [unwired: 1 in, 2 out]
        n282 = Or(x="Vertical scroll bar", y="Horizontal scroll bar") -> (x .or. y?=w605:bool)
        n283 = Bundle By Name(cluster=w616, "Bar?"=w605) -> (w606:T4)
      }
      frame "Load Picture" {
        n284 = Unbundle By Name(w644) -> ("Chart Select"=w626:refnum<vi>, "Queue.Data Path"=w634:path, "Picture"=w620:refnum<vi>)
        n285 = property class="Pict"(reference=w620, "Value"=picture data[5B] ("值")) -> ()  [unwired: 1 in, 2 out]
        n286 = Build Path(base path=w634, name or relative path=path "Config.ini" ("名称或相对路径")) -> (appended path=w638:path)
        n287 = List Folder(path=w634) -> (folder names=w625:string[])  [unwired: 3 in, 3 out]
        n288 = call <vilib>:"Open Config Data.vi"("configuration file path"=w638) -> ("error out"=w642:errorcluster, "refnum"=w643:T15)  [unwired: 8 in, 1 out]
        n289 = call-poly <vilib>:"Read Key.vi"("section"="FlowChart", "error in (no error)"=w642, "key"="Current_Picture", "refnum"=w643) -> ("error out"=w640:errorcluster, "value"=w633:string, "refnum out"=w641:T15)  [unwired: 4 in, 1 out]
        n290 = Bundle By Name(cluster=w644, "PictureList"=w625) -> (w630:T4)
        n291 = call <vilib>:"Close Config Data.vi"("error in (no error)"=w640, "refnum"=w641) -> ()  [unwired: 8 in, 2 out]
        n292 = Search 1D Array(1D array=w625, element=w633) -> (index of element=w623:i32)  [unwired: 1 in]
        n293 = Index Array(array=w625) -> (element=w632:string)  [unwired: 1 in]
        n294 = Greater Or Equal To 0?(x=w623) -> (x >= 0?=w624:bool)
        n295 = Unbundle By Name(w630) -> ("Queue.Data Path"=w629:path)
        n296 = Select(t=w623, s=w624, f=0) -> (s? t:f=w621:i32)
        n297 = property class="Ring"(reference=w626, "Strings []"=w625, "Value"=w621) -> ()  [unwired: 1 in, 2 out]
        n298 = Select(t=w633, s=w624, f=w632) -> (s? t:f=w631:string)
        n299 = case shown="默认" w631 {
          selector: w631 -> [w648 _]
          tunnel: [w658 w682] -> w635
          tunnel: w630 -> [w649 w682]
          tunnel: w629 -> [w657 _]
          tunnel: "%s.png" ("格式字符串") -> [w654 _]
          tunnel: [w647 _] -> w627
          frame Default {
            n300 = Build Path(base path=w657, name or relative path=w648) -> (appended path=w656:path)
            n301 = Format Into String(format string=w654, w648) -> (resulting string=w655:string)  [unwired: 2 in, 1 out]
            n302 = Build Path(base path=w656, name or relative path=w655) -> (appended path=w653:path)
            n303 = call <vilib>:"Check if File or Folder Exists.vi"("path"=w653) -> ("error out"=w650:errorcluster, "file or folder exists?"=w652:bool, "dup path"=w651:path)  [unwired: 8 in]
            n304 = case shown="真" w652 {
              tunnel: [w659 w681] -> w658
              tunnel: w649 -> [w659 w680]
              tunnel: w651 -> [_ w669]
              tunnel: w650 -> [_ w668]
              tunnel: w649 -> [_ w667]
              tunnel: w648 -> [_ w663]
              tunnel: [_ "Panel Change"] -> w647
              frame False {
              }
              frame True {
                n305 = call <vilib>:"Read PNG File.vi"("error in (no error)"=w668, "path to PNG file"=w669) -> ("image data"=w679:T18)  [unwired: 7 in, 2 out]
                n306 = Bundle By Name(cluster=w680, "CPicture"=w663) -> (w664:T4)
                n307 = Unbundle By Name(w667) -> ("Queue.Data"=w666:refnum<queue>)
                n308 = call <vilib>:"Draw Flattened Pixmap.vi"("image data"=w679) -> ("new picture"=w662:picture)  [unwired: 8 in]
                n309 = call <vilib>:"Picture to Pixmap.vi"("picture"=w662) -> ("image data"=w678:T18)  [unwired: 9 in, 1 out]
                n310 = Unbundle By Name(w678) -> ("Rectangle.right"=w676:i16, "Rectangle.left"=w675:i16, "Rectangle.bottom"=w674:i16, "Rectangle.top"=w673:i16)
                n311 = call "Queue In.vi"("Data"=w663, "Message"="Load Config", "Queue In"=w666) -> ()  [unwired: 7 in, 2 out]
                n312 = Subtract(x=w676, y=w675) -> (x-y=w672:i16)
                n313 = Subtract(x=w674, y=w673) -> (x-y=w671:i16)
                n314 = Bundle By Name(cluster=T3 {"Width"=0, "Height"=0} ("绘图区域大小"), "Width"=w672, "Height"=w671) -> (w661:T3)
                n315 = Bundle By Name(cluster=w664, "Area"=w661) -> (w681:T4)
                n316 = Unbundle By Name(w681) -> ("Picture"=w670:refnum<vi>)
                n317 = property on="属性节点" class="Pict"(reference=w670, "Value"=w662, "Draw Area Size"=w661) -> ()  [unwired: 1 in, 2 out]
              }
            }
          }
          frame "" {
          }
        }
      }
      frame "WorkMode" {
        n318 = in-place {
          in-place-border: w684 -> [w690]
          n319 = in-place-cluster #13(w685) -> ("WorkMode.Mode"=w689:string)
          n320 = Variant To Data(type=w689, Variant=w690) -> (data=w688:string)  [unwired: 1 in, 1 out]
          n321 = in-place-cluster #13("WorkMode.Mode"=w688) -> (w683:T4)
        }
      }
      frame "Mode Change" {
        n322 = in-place {
          in-place-border: w696 -> [w702]
          n323 = in-place-cluster #14(w697) -> ("WorkMode.Data"=w701:string)
          n324 = Variant To Data(type=w701, Variant=w702) -> (data=w700:string)  [unwired: 1 in, 1 out]
          n325 = in-place-cluster #14("WorkMode.Data"=w700) -> (w695:T4)
        }
        n326 = Unbundle By Name(w695) -> ("WorkMode.Data"=w694:string)
        n327 = Fract/Exp String To Number(string=w694) -> (number=w693:dbl)  [unwired: 3 in, 1 out]
        n328 = Greater Than 0?(x=w693) -> (x > 0?=w691:bool)
        n329 = Bundle By Name(cluster=w695, "WorkMode.Mode?"=w691) -> (w692:T4)
      }
      frame "WorkMode Edit" {
        n330 = Unbundle By Name(w703) -> ("WorkMode.Mode"=w708:string, "Queue.Project Name"=w707:string)
        n331 = call "FlowChart Edit.vi"("Name"=w707, "Identifier In"=w708) -> ("OK？"=w704:bool, "Identifier Out"=w705:string)  [unwired: 6 in, 2 out]
        n332 = case shown="真" w704 {
          tunnel: w703 -> [w711 w718]
          tunnel: [w711 w717] -> w706
          tunnel: w705 -> [_ w716]
          tunnel: w703 -> [_ w715]
          frame False {
          }
          frame True {
            n333 = Unbundle By Name(w715) -> ("Queue.Data"=w714:refnum<queue>, "WorkMode.Mode"=w713:string)
            n334 = Bundle By Name(cluster=w718, "WorkMode.Mode"=w716) -> (w717:T4)
            n335 = call "Queue In.vi"("Data"=w713, "Message"="WorkMode", "Queue In"=w714) -> ()  [unwired: 7 in, 2 out]
          }
        }
      }
      frame "ShowLable" {
        n336 = flat-sequence {
          tunnel: w721 -> [w730]
          tunnel: [w730] -> w722
          tunnel: w721 -> [w726]
          tunnel: [w725] -> w719
          tunnel: w722 -> [w734]
          tunnel: [w731] -> w720
          tunnel: w719 -> [w731]
          tunnel: w720 -> [w741]
          frame #0 {
            n337 = Unbundle By Name(w726) -> ("Queue.VI"=w729:refnum<vi>)
            n338 = property class="VI"(reference=w729) -> ("Panel"=w728:refnum<vi>)  [unwired: 1 in, 2 out]
            n339 = property class="Pnl"(reference=w728, "DeferPanUpdts"=TRUE ("延迟前面板更新")) -> (reference out=w725:refnum<vi>)  [unwired: 1 in, 1 out]
          }
          frame #1 {
            n340 = Unbundle By Name(w734) -> ("Type"=w733:map{string, map{string, refnum<vi>}})
            n341 = for {
              tunnel: w733 -> [w737] mode=indexing
              tunnel: "ShowLable" -> [w735]
              n342 = Unbundle By Name(w737) -> ("Control"=w736:map{string, refnum<vi>})
              n343 = for {
                tunnel: w736 -> [w740] mode=indexing
                tunnel: w735 -> [w738]
                n344 = Unbundle By Name(w740) -> ("Ref"=w739:refnum<vi>)
                n345 = property class="Ctl"(reference=w739, "Caption.Visible"=w738) -> ()  [unwired: 1 in, 2 out]
              }
            }
          }
          frame #2 {
            n346 = property class="Pnl"(reference=w741, "DeferPanUpdts"=FALSE ("延迟前面板更新")) -> ()  [unwired: 1 in, 2 out]
          }
        }
      }
      frame "Write Prepare" {
        n347 = Unbundle By Name(w743) -> ()  [unwired: 1 out]
        n348 = case shown="真" TRUE {
          tunnel: w745 -> [_ w758]
          tunnel: w743 -> [_ w749]
          frame False {
          }
          frame True {
            n349 = Variant To Data(type=cluster{"Name":string, "Data":string} {"Name"="", "Data"=""} ("Set"), Variant=w758) -> (data=w756:cluster{"Name":string, "Data":string})  [unwired: 1 in, 1 out]
            n350 = Unbundle By Name(w756) -> ("Name"=w748:string, "Data"=w752:string)
            n351 = Equal?(x=w752, y="1") -> (x = y?=w750:bool)
            n352 = call <vilib>:"Delimited String to 1D String Array.vi"("delimiter"=" ", "delimited string"=w748) -> ("string array"=w754:string[])  [unwired: 9 in]
            n353 = Index Array(array=w754) -> (element=w753:string)  [unwired: 1 in]
            n354 = case shown="\"Bump\", \"HVFS\", \"HValve\", \"VVFS\", \"VValve\"" w753 {
              selector: w753 -> [_ w767]
              tunnel: w750 -> [_ w761]
              tunnel: w749 -> [_ w762]
              tunnel: w748 -> [_ w765]
              frame Default {
              }
              frame "Bump", "HVFS", "HValve", "VVFS", "VValve" {
                n355 = Unbundle By Name(w762) -> ("Type"=w768:map{string, map{string, refnum<vi>}})
                n356 = Look In Map(map=w768, key=w767) -> (value=w766:map{string, refnum<vi>})  [unwired: 1 in, 1 out]
                n357 = Look In Map(map=w766, key=w765) -> (value=w764:refnum<vi>)  [unwired: 1 in, 1 out]
                n358 = property class="Ctl"(reference=w764) -> ("TipStrip"=w759:string, "Desc"=w760:string)  [unwired: 1 in, 2 out]
                n359 = Select(t="打开", s=w761, f="关闭") -> (s? t:f=w769:string)
                n360 = Format Into String(format string="确定%s“%s”?" ("消息"), w769, w759) -> (resulting string=w772:string)  [unwired: 2 in, 1 out]
                n361 = Two Button Dialog(message=w772) -> (T button?=w763:bool)  [unwired: 2 in]
                n362 = case shown="真" w763 {
                  tunnel: w762 -> [_ w777]
                  tunnel: w761 -> [_ w783]
                  tunnel: w760 -> [_ w781]
                  tunnel: w759 -> [_ w779]
                  frame False {
                  }
                  frame True {
                    n363 = call "000_Bool True.vi"("Value"=w783) -> ("String Out"=w778:string)  [unwired: 8 in, 2 out]
                    n364 = Unbundle By Name(w777) -> ("Queue.Caller"=w782:refnum<queue>)
                    n365 = Unbundle By Name(w777) -> ("Queue.Data"=w776:refnum<queue>)
                    n366 = Format Into String(format string="%s-->%s" ("格式字符串"), w779, w778) -> (resulting string=w775:string)  [unwired: 2 in, 1 out]
                    n367 = call "000_Source Write.vim"("Data"=w778, "Name"=w781, "Queue In"=w782) -> ()  [unwired: 6 in, 3 out]
                    n368 = call "Queue In.vi"("Data"=w775, "Message"="Log", "Queue In"=w776) -> ()  [unwired: 7 in, 2 out]
                  }
                }
              }
            }
          }
        }
      }
      frame "LogRead" {
        n369 = Unbundle By Name(w785) -> ()  [unwired: 1 out]
        n370 = One Button Dialog(message="暂无日志" ("消息")) -> ()  [unwired: 1 in, 1 out]
      }
      frame "FlowChartEdit" {
        n371 = Unbundle By Name(w797) -> ("Queue.Data Path"=w796:path, "CPicture"=w793:string)
        n372 = Build Path(base path=w796, name or relative path=w793) -> (appended path=w795:path)
        n373 = Format Into String(format string="%s.csv" ("格式字符串"), w793) -> (resulting string=w792:string)  [unwired: 2 in, 1 out]
        n374 = Build Path(base path=w795, name or relative path=w792) -> (appended path=w791:path)
        n375 = call <vilib>:"Check if File or Folder Exists.vi"("path"=w791) -> ("error out"=w788:errorcluster, "file or folder exists?"=w790:bool, "dup path"=w789:path)  [unwired: 8 in]
        n376 = case shown="真" w790 {
          tunnel: w789 -> [_ w801]
          tunnel: w788 -> [_ w800]
          frame False {
          }
          frame True {
            n377 = call <vilib>:"Show in File System.vi"("error in (no error)"=w800, "file or directory path"=w801) -> ()  [unwired: 9 in, 1 out]
          }
        }
      }
      frame "Panel Change" {
        n378 = Unbundle By Name(w805) -> ("Bar?"=w802:bool, "Panel"=w804:refnum<vi>, "Area"=w803:T3)
        n379 = case shown="假" w802 {
          tunnel: w804 -> [w815 _]
          tunnel: w803 -> [w813 _]
          frame False {
            n380 = property class="Pane"(reference=w815) -> (reference out=w811:refnum<vi>, "Bounds"=w814:T3)  [unwired: 1 in, 1 out]
            n381 = Subtract(x=w814, y=w813) -> (x-y=w812:T3)
            n382 = To Word Integer(number=w812) -> (16bit integer=w809:cluster{"Width":i16, "Height":i16})
            n383 = expression code="-x/2"(w809) -> (w810:cluster{"Width":i16, "Height":i16})
            n384 = To Word Integer(number=w810) -> (16bit integer=w808:cluster{"Width":i16, "Height":i16})
            n385 = property class="Pane"(reference=w811, "Origin"=w808) -> ()  [unwired: 1 in, 2 out]
          }
          frame True {
          }
        }
      }
      frame "Picture Add" {
        n386 = call "文件对话框"("pattern (all files)"="*.png") -> ("selected path"=w817:path, "exists"=w819:bool, "cancelled"=w816:bool, "error out"=w818:errorcluster)  [unwired: 11 in]
        n387 = case shown="无错误" w818 {
          selector: w818 -> [w825 _]
          tunnel: w819 -> [w830 _]
          tunnel: w817 -> [w829 _]
          tunnel: w816 -> [w828 _]
          tunnel: w822 -> [w827 w869]
          tunnel: [w826 w869] -> w821
          frame No Error {
            n388 = case shown="真" w830 {
              tunnel: w829 -> [_ w835]
              tunnel: w828 -> [_ w836]
              tunnel: w827 -> [w831 w834]
              tunnel: [w831 w833] -> w826
              tunnel: w825 -> [_ w832]
              frame False {
              }
              frame True {
                n389 = case shown="假" w836 {
                  tunnel: w835 -> [w849 _]
                  tunnel: w834 -> [w843 w868]
                  tunnel: [w842 w868] -> w833
                  tunnel: w832 -> [w848 _]
                  frame False {
                    n390 = Unbundle By Name(w843) -> ("Queue.Data Path"=w847:path)
                    n391 = call <vilib>:"Get File Extension.vi"("error in (no error)"=w848, "file"=w849) -> ("filename without extension"=w838:string, "dup file"=w844:path)  [unwired: 5 in, 3 out]
                    n392 = List Folder(path=w847) -> (path out=w845:path, folder names=w841:string[])  [unwired: 3 in, 2 out]
                    n393 = Search 1D Array(1D array=w841, element=w838) -> (index of element=w846:i32)  [unwired: 1 in]
                    n394 = Less Than 0?(x=w846) -> (x < 0?=w840:bool)
                    n395 = case shown="假" w840 {
                      tunnel: "\"%s\"已存在，是否替换？" ("格式字符串") -> [w866 _]
                      tunnel: w838 -> [w865 _]
                      tunnel: [w863 TRUE ("T button?")] -> w837
                      frame False {
                        n396 = Format Into String(initial string=w866, w865) -> (resulting string=w864:string)  [unwired: 2 in, 1 out]
                        n397 = Two Button Dialog(message=w864) -> (T button?=w863:bool)  [unwired: 2 in]
                      }
                      frame True {
                      }
                    }
                    n398 = case shown="假" w837 {
                      tunnel: w845 -> [_ w862]
                      tunnel: w844 -> [_ w861]
                      tunnel: w843 -> [w850 w860]
                      tunnel: [w850 w859] -> w842
                      tunnel: w838 -> [_ w851]
                      frame False {
                      }
                      frame True {
                        n399 = Build Path(base path=w862, name or relative path=w851) -> (appended path=w858:path)
                        n400 = Strip Path(path=w861) -> (name=w857:string)  [unwired: 1 out]
                        n401 = Create Folder(path (use dialog)=w858) -> (created path=w855:path)  [unwired: 2 in, 2 out]
                        n402 = Build Path(base path=w855, name or relative path=w857) -> (appended path=w856:path)
                        n403 = Unbundle By Name(w860) -> ("Queue.Data"=w854:refnum<queue>)
                        n404 = Copy(9:TRUE ("覆盖(F)"), 10:w856, 11:w861) -> ()  [unwired: 2 in, 3 out]
                        n405 = call "Queue In.vi"("Data"=w851, "Message"="Load Config,Save Config,Load Picture", "Queue In"=w854) -> ()  [unwired: 7 in, 2 out]
                        n406 = Bundle By Name(cluster=w860, "CPicture"=w851) -> (w859:T4)
                      }
                    }
                  }
                  frame True {
                  }
                }
              }
            }
          }
          frame Error {
          }
        }
      }
      frame "Picture Delete" {
        n407 = Unbundle By Name(w872) -> ("CPicture"=w875:string)
        n408 = Format Into String(format string="您所编辑的全部数据将消失！确定要删除\"%s\"吗?" ("消息"), w875) -> (resulting string=w874:string)  [unwired: 2 in, 1 out]
        n409 = Two Button Dialog(message=w874) -> (T button?=w873:bool)  [unwired: 2 in]
        n410 = case shown="真" w873 {
          tunnel: w872 -> [w879 w887]
          tunnel: [w879 w887] -> w871
          tunnel: [_ "Load Picture"] -> w870
          frame False {
          }
          frame True {
            n411 = Unbundle By Name(w887) -> ("Queue.Data Path"=w886:path, "CPicture"=w885:string)
            n412 = Build Path(base path=w886, name or relative path=w885) -> (appended path=w884:path)
            n413 = call <vilib>:"Check if File or Folder Exists.vi"("path"=w884) -> ("error out"=w881:errorcluster, "file or folder exists?"=w883:bool, "dup path"=w882:path)  [unwired: 8 in]
            n414 = case shown="真" w883 {
              tunnel: w882 -> [_ w890]
              tunnel: w881 -> [_ w889]
              frame False {
              }
              frame True {
                n415 = Delete(path (use dialog)=w890, entire hierarchy (F)=TRUE ("整个层次结构(F)"), error in=w889) -> ()  [unwired: 2 in, 3 out]
              }
            }
          }
        }
      }
      frame "Control Hide" {
        n416 = Variant To Data(type=refnum<vi> refnum ("引用输出"), Variant=w896) -> (data=w894:refnum<vi>)  [unwired: 1 in, 1 out]
        n417 = property class="Ctl"(reference=w894) -> (reference out=w891:refnum<vi>, "TipStrip"=w893:string, "Label.Text"=w892:string)  [unwired: 1 in, 1 out]
        n418 = Format Into String(format string="确定要删除吗“%s”？" ("格式字符串"), w893) -> (resulting string=w900:string)  [unwired: 2 in, 1 out]
        n419 = Two Button Dialog(message=w900) -> (T button?=w899:bool)  [unwired: 2 in]
        n420 = case shown="真" w899 {
          tunnel: w897 -> [_ w908]
          tunnel: w892 -> [_ w905]
          tunnel: w891 -> [_ w904]
          frame False {
          }
          frame True {
            n421 = Unbundle By Name(w908) -> ("Queue.Data"=w907:refnum<queue>)
            n422 = property class="Ctl"(reference=w904, "Visible"=FALSE ("可见")) -> ()  [unwired: 1 in, 2 out]
            n423 = call "Queue In.vi"("Data"=w905, "Message"="Hide", "Queue In"=w907) -> ()  [unwired: 7 in, 2 out]
          }
        }
      }
      frame "Chart Select" {
        n424 = flat-sequence {
          tunnel: w912 -> [w919]
          tunnel: [w916] -> w910
          tunnel: [w915] -> w909
          tunnel: [w923] -> w911
          tunnel: w910 -> [w923]
          tunnel: w909 -> [w920]
          frame #0 {
            n425 = Unbundle By Name(w919) -> ("PictureList"=w918:string[])
            n426 = Index Array(array=w918, index="Chart Select") -> (element=w915:string)
            n427 = Bundle By Name(cluster=w919, "CPicture"=w915) -> (w916:T4)
          }
          frame #1 {
            n428 = Unbundle By Name(w923) -> ("Queue.Data"=w922:refnum<queue>)
            n429 = call "Queue In.vi"("Data"=w920, "Message"="Load Config,Save Config,Load Picture", "Queue In"=w922) -> ()  [unwired: 7 in, 2 out]
          }
        }
      }
      frame "Control Refer" {
        n430 = in-place {
          in-place-border: w930 -> [w953]
          n431 = in-place-cluster #15(w931) -> ("Property"=w952:T13)
          n432 = Variant To Data(type=w952, Variant=w953) -> (data=w951:T13)  [unwired: 1 in, 1 out]
          n433 = in-place-cluster #15("Property"=w951) -> (w929:T4)
        }
        n434 = Unbundle By Name(w929) -> ("Type"=w927:map{string, map{string, refnum<vi>}}, "Property"=w928:T13)
        n435 = for {
          tunnel: w928 -> [w940] mode=indexing
          shift-right: [w941] -> w924
          shift-left: w927 -> [w942]
          n436 = Unbundle By Name(w940) -> ("Control"=w936:string, "Data.Ref"=w935:refnum<vi>)
          n437 = call <vilib>:"Delimited String to 1D String Array.vi"("delimiter"=" ", "delimited string"=w936) -> ("string array"=w938:string[])  [unwired: 9 in]
          n438 = Index Array(array=w938) -> (element=w937:string)  [unwired: 1 in]
          n439 = in-place {
            in-place-border: w936 -> [w946]
            in-place-border: w935 -> [w945]
            in-place-border: LVMapReplaceAction."Add or Modify Entry" ("操作") -> [w944]
            n440 = in-place-map #16(w942, w937) -> (w948:map{string, refnum<vi>})  [unwired: 1 in, 1 out]
            n441 = in-place {
              in-place-border: w945 -> [w950]
              in-place-border: w944 -> [w949]
              in-place-border: [w949] -> w943
              n442 = in-place-map #17(w948, w946) -> ()  [unwired: 1 in, 2 out]
              n443 = in-place-map #17(w950, w949) -> (w947:map{string, refnum<vi>})  [unwired: 2 out]
            }
            n444 = in-place-map #16(w947, w943) -> (w941:map{string, map{string, refnum<vi>}})  [unwired: 2 out]
          }
        }
        n445 = Bundle By Name(cluster=w929, "Type"=w924) -> (w926:T4)
        n446 = Unbundle By Name(w926) -> ("UE"=w925:refnum<user-event>)
        n447 = Generate User Event(user event=w925, event data cluster=w924) -> ()  [unwired: 2 in, 2 out]
      }
      frame "Control Edit" {
        n448 = Variant To Data(type=refnum<vi> refnum ("引用输出"), Variant=w963) -> (data=w961:refnum<vi>)  [unwired: 1 in, 1 out]
        n449 = Unbundle By Name(w964) -> ("Queue.Data"=w956:refnum<queue>, "Queue.Project Name"=w955:string)
        n450 = property class="Ctl"(reference=w961) -> (reference out=w958:refnum<vi>, "Desc"=w954:string)  [unwired: 1 in, 1 out]
        n451 = call "FlowChart Edit.vi"("Name"=w955, "Identifier In"=w954) -> ("OK？"=w960:bool, "Tips"=w959:string, "Identifier Out"=w957:string)  [unwired: 6 in, 1 out]
        n452 = case shown="真" w960 {
          tunnel: w959 -> [_ w971]
          tunnel: w958 -> [_ w972]
          tunnel: w957 -> [_ w970]
          tunnel: w956 -> [_ w969]
          frame False {
          }
          frame True {
            n453 = property class="Ctl"(reference=w972, "Desc"=w970, "TipStrip"=w971) -> ("Label.Text"=w967:string)  [unwired: 1 in, 2 out]
            n454 = call "Queue In.vi"("Data"=w967, "Message"="ID Change", "Queue In"=w969) -> ()  [unwired: 7 in, 2 out]
          }
        }
      }
      frame "Refresh" {
      }
      frame "====System====" {
      }
      frame "Refresh Class Ref" {
        n455 = case shown="\"Refresh Class Ref\"" w979 {
          tunnel: w982 -> [w985 w988]
          tunnel: [w985 w987] -> w981
          tunnel: w980 -> [_ w986]
          frame "eee", Default {
          }
          frame "Refresh Class Ref" {
            n456 = in-place {
              in-place-border: w986 -> [w991]
              n457 = in-place-cluster #18(w988) -> ("Queue"=w990:T1)
              n458 = Variant To Data(type=w990, Variant=w991) -> (data=w989:T1)  [unwired: 1 in, 1 out]
              n459 = in-place-cluster #18("Queue"=w989) -> (w987:T4)
            }
          }
        }
      }
      frame "Exit" {
        n460 = Unbundle By Name(w993) -> ("Queue.Message"=w997:refnum<queue>, "Queue.Data"=w996:refnum<queue>, "Queue.UE"=w992:refnum<user-event>)
        n461 = Build Array(w997, w996) -> (w995:refnum<queue>[])
        n462 = Generate User Event(user event=w992, event data cluster=w994) -> ()  [unwired: 2 in, 2 out]
        n463 = for {
          tunnel: w995 -> [w1004] mode=indexing
          tunnel: w994 -> [w1003]
          n464 = call "Queue In.vi"("Message"=w1003, "Queue In"=w1004) -> ()  [unwired: 8 in, 2 out]
        }
        n465 = call "Queue Clear.vi"("error in (no error)"=w999, "Queue In"=w1001) -> ("error out"=w998:errorcluster, "Queue Out"=w1000:refnum<queue>)  [unwired: 8 in]
      }
      frame "Quit" {
      }
    }
    n466 = call "Queue In.vi"("error in (no error)"=w581, "Data"=w579, "Message"=w580, "Queue In"=w584) -> ("error out"=w582:errorcluster, "Queue Out"=w583:refnum<queue>)  [unwired: 6 in]
  }
  n467 = call "000 Driver Message.vi"("Queue In"=w3) -> ("error out"=w13:errorcluster)  [unwired: 8 in, 2 out]
  n468 = call "Queue Release.vi"("error in (no error)"=w16, "Queue In"=w17) -> ("error out"=w14:errorcluster)  [unwired: 9 in]
  n469 = call "Queue Release.vi"("error in (no error)"=w24, "Queue In"=w25) -> ("error out"=w21:errorcluster)  [unwired: 9 in]
  n470 = Unregister For Events(event registration refnum=w27) -> (error out=w26:errorcluster)  [unwired: 1 in]
  n471 = Destroy User Event(user event=w12, error in=w26) -> (error out=w22:errorcluster)
  n472 = Call Chain() -> (call chain=w19:string[])
  n473 = Merge Errors(w22, w21, w13, w14) -> (w20:errorcluster)
  n474 = Array Size(array=w19) -> (size(s)=w18:i32)
  n475 = case shown="2.." w18 {
    tunnel: w20 -> [_ w1009]
    frame 0, Default {
    }
    frame 2.. {
      n476 = invoke class="VI" method="FP.Close"(error in=w1009) -> ()  [unwired: 2 in, 3 out]
    }
  }
